vi "myRIO_BRig_Host_endExp_storeFiles__v4.vi"(0 "input_filePath":path) -> ()   [LabVIEW 2014]
panel:
  out "error2":errorcluster
  out "error1":errorcluster
  in  "input_error":errorcluster
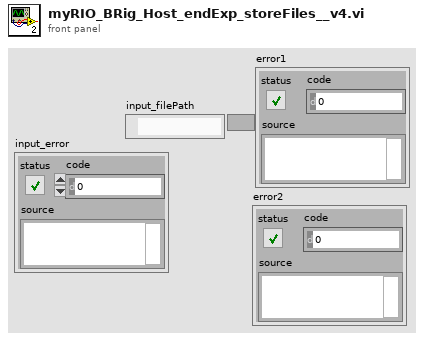
[diagram p1: front panel]
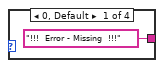
[diagram p2: hidden frame]
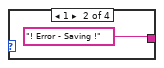
[diagram p3: hidden frame]
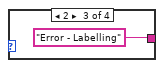
[diagram p4: hidden frame]
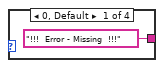
[diagram p5: hidden frame]
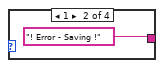
[diagram p6: hidden frame]
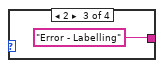
[diagram p7: hidden frame]
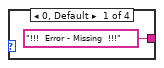
[diagram p8: hidden frame]
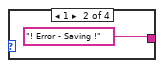
[diagram p9: hidden frame]
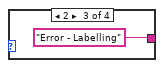
[diagram p10: hidden frame]
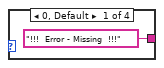
[diagram p11: hidden frame]
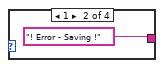
[diagram p12: hidden frame]
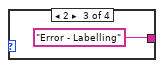
[diagram p13: hidden frame]
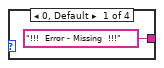
[diagram p14: hidden frame]
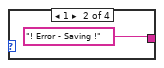
[diagram p15: hidden frame]
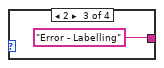
[diagram p16: hidden frame]
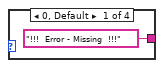
[diagram p17: hidden frame]
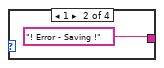
[diagram p18: hidden frame]
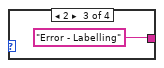
[diagram p19: hidden frame]
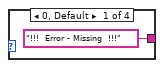
[diagram p20: hidden frame]
diagram:
  w2 = "\r"
  # "Workbooks"
  # "Application"
  # "Is Excel Running?"
  n1 = flat-sequence {
    tunnel: "input_filePath" -> [w403]
    tunnel: "input_error" -> [w400]
    tunnel: [w399] -> w395
    tunnel: [w402] -> w394
    tunnel: [w401] -> w393
    tunnel: [w398] -> w391
    tunnel: w395 -> [w446]
    tunnel: w394 -> [w447]
    tunnel: w393 -> [w407]
    tunnel: [w447] -> w392
    tunnel: w391 -> [w406]
    tunnel: [w446] -> w390
    tunnel: [w442] -> w389
    tunnel: [w441] -> w388
    tunnel: [w437] -> w314
    tunnel: [w436] -> w307
    tunnel: [w433] -> w279
    tunnel: [w430] -> w278
    tunnel: [w429] -> w277
    tunnel: [w428] -> w276
    tunnel: [w422] -> w268
    tunnel: [w421] -> w267
    tunnel: [w417] -> w266
    tunnel: [w416] -> w265
    tunnel: [w412] -> w264
    tunnel: [w411] -> w263
    tunnel: [w405] -> w40
    tunnel: [w404] -> w39
    tunnel: w392 -> [w489]
    tunnel: w390 -> [w485]
    tunnel: w389 -> [w484]
    tunnel: w388 -> [w488]
    tunnel: [w489] -> w387
    tunnel: [w487] -> w386
    tunnel: [w486] -> w385
    tunnel: [w450] -> w384
    tunnel: [w484] -> w383
    tunnel: [w483] -> w315
    tunnel: w314 -> [w483]
    tunnel: [w481] -> w308
    tunnel: w307 -> [w482]
    tunnel: [w480] -> w306
    tunnel: w279 -> [w478]
    tunnel: w278 -> [w477]
    tunnel: w277 -> [w465]
    tunnel: w276 -> [w467]
    tunnel: [w478] -> w270
    tunnel: w268 -> [w476]
    tunnel: w267 -> [w469]
    tunnel: w266 -> [w475]
    tunnel: w265 -> [w471]
    tunnel: w264 -> [w474]
    tunnel: w263 -> [w473]
    tunnel: [w464] -> w257
    tunnel: [w477] -> w251
    tunnel: [w466] -> w245
    tunnel: [w476] -> w239
    tunnel: [w468] -> w233
    tunnel: [w475] -> w227
    tunnel: [w470] -> w221
    tunnel: [w474] -> w215
    tunnel: [w472] -> w209
    tunnel: [w458] -> w208
    tunnel: [w457] -> w198
    tunnel: [w456] -> w190
    tunnel: [w455] -> w184
    tunnel: [w454] -> w179
    tunnel: [w453] -> w41
    tunnel: w40 -> [w453]
    tunnel: w39 -> [w452]
    tunnel: [w449] -> w38
    tunnel: [w448] -> w35
    tunnel: w387 -> [w531]
    tunnel: w386 -> [w529]
    tunnel: w385 -> [w528]
    tunnel: w384 -> [w495]
    tunnel: w383 -> [w530]
    tunnel: [w531] -> w370
    tunnel: [w530] -> w368
    tunnel: [w529] -> w366
    tunnel: [w528] -> w364
    tunnel: [w527] -> w362
    tunnel: [w522] -> w360
    tunnel: [w524] -> w316
    tunnel: w315 -> [w524]
    tunnel: [w525] -> w309
    tunnel: w308 -> [w525]
    tunnel: w306 -> [w526]
    tunnel: [w526] -> w305
    tunnel: [w523] -> w301
    tunnel: [w519] -> w271
    tunnel: w270 -> [w519]
    tunnel: [w520] -> w258
    tunnel: w257 -> [w520]
    tunnel: [w515] -> w252
    tunnel: w251 -> [w515]
    tunnel: [w516] -> w246
    tunnel: w245 -> [w516]
    tunnel: [w506] -> w240
    tunnel: w239 -> [w506]
    tunnel: [w509] -> w234
    tunnel: w233 -> [w509]
    tunnel: [w505] -> w228
    tunnel: w227 -> [w505]
    tunnel: [w508] -> w222
    tunnel: w221 -> [w508]
    tunnel: [w504] -> w216
    tunnel: w215 -> [w504]
    tunnel: [w507] -> w210
    tunnel: w209 -> [w507]
    tunnel: w208 -> [w521]
    tunnel: [w521] -> w204
    tunnel: [w518] -> w203
    tunnel: w198 -> [w517]
    tunnel: [w517] -> w196
    tunnel: [w514] -> w193
    tunnel: [w513] -> w191
    tunnel: w190 -> [w510]
    tunnel: [w510] -> w185
    tunnel: w184 -> [w511]
    tunnel: [w511] -> w180
    tunnel: w179 -> [w512]
    tunnel: [w512] -> w175
    tunnel: [w503] -> w174
    tunnel: [w502] -> w169
    tunnel: [w501] -> w164
    tunnel: [w500] -> w155
    tunnel: [w499] -> w153
    tunnel: [w498] -> w151
    tunnel: [w497] -> w149
    tunnel: [w496] -> w147
    tunnel: [w494] -> w42
    tunnel: w41 -> [w494]
    tunnel: w38 -> [w493]
    tunnel: [w493] -> w36
    tunnel: w35 -> [w492]
    tunnel: [w492] -> w33
    tunnel: [w491] -> w32
    tunnel: [w490] -> w31
    tunnel: w370 -> [w639]
    tunnel: [w639] -> w369
    tunnel: w368 -> [w638]
    tunnel: [w638] -> w367
    tunnel: w366 -> [w637]
    tunnel: [w637] -> w365
    tunnel: w364 -> [w636]
    tunnel: [w636] -> w363
    tunnel: w362 -> [w634]
    tunnel: [w634] -> w361
    tunnel: w360 -> [w635]
    tunnel: [w635] -> w359
    tunnel: [w630] -> w317
    tunnel: w316 -> [w630]
    tunnel: [w629] -> w310
    tunnel: w309 -> [w629]
    tunnel: w305 -> [w628]
    tunnel: [w628] -> w304
    tunnel: w301 -> [w627]
    tunnel: [w627] -> w300
    tunnel: [w626] -> w272
    tunnel: w271 -> [w626]
    tunnel: [w625] -> w259
    tunnel: w258 -> [w625]
    tunnel: [w624] -> w253
    tunnel: w252 -> [w624]
    tunnel: [w623] -> w247
    tunnel: w246 -> [w623]
    tunnel: [w622] -> w241
    tunnel: w240 -> [w622]
    tunnel: [w621] -> w235
    tunnel: w234 -> [w621]
    tunnel: [w620] -> w229
    tunnel: w228 -> [w620]
    tunnel: [w619] -> w223
    tunnel: w222 -> [w619]
    tunnel: [w618] -> w217
    tunnel: w216 -> [w618]
    tunnel: [w617] -> w211
    tunnel: w210 -> [w617]
    tunnel: [w616] -> w205
    tunnel: w204 -> [w616]
    tunnel: w203 -> [w615]
    tunnel: [w615] -> w199
    tunnel: [w614] -> w197
    tunnel: w196 -> [w614]
    tunnel: w193 -> [w606]
    tunnel: [w613] -> w192
    tunnel: w191 -> [w613]
    tunnel: [w612] -> w186
    tunnel: w185 -> [w612]
    tunnel: [w611] -> w181
    tunnel: w180 -> [w611]
    tunnel: [w610] -> w176
    tunnel: w175 -> [w610]
    tunnel: w174 -> [w609]
    tunnel: [w609] -> w170
    tunnel: w169 -> [w608]
    tunnel: [w608] -> w165
    tunnel: w164 -> [w607]
    tunnel: [w607] -> w160
    tunnel: [w606] -> w156
    tunnel: w155 -> [w605]
    tunnel: [w605] -> w154
    tunnel: w153 -> [w604]
    tunnel: [w604] -> w152
    tunnel: w151 -> [w603]
    tunnel: [w603] -> w150
    tunnel: w149 -> [w602]
    tunnel: [w602] -> w148
    tunnel: w147 -> [w601]
    tunnel: [w601] -> w146
    tunnel: [w600] -> w43
    tunnel: w42 -> [w600]
    tunnel: [w599] -> w37
    tunnel: w36 -> [w599]
    tunnel: [w598] -> w34
    tunnel: w33 -> [w598]
    tunnel: w32 -> [w596]
    tunnel: w31 -> [w597]
    tunnel: [w597] -> w30
    tunnel: [w596] -> w27
    tunnel: w369 -> [w704]
    tunnel: w367 -> [w703]
    tunnel: w365 -> [w701]
    tunnel: w363 -> [w700]
    tunnel: w361 -> [w702]
    tunnel: w359 -> [w697]
    tunnel: [w704] -> w382
    tunnel: [w703] -> w381
    tunnel: [w702] -> w380
    tunnel: [w684] -> w379
    tunnel: [w699] -> w378
    tunnel: [w698] -> w377
    tunnel: [w696] -> w318
    tunnel: w317 -> [w696]
    tunnel: [w692] -> w311
    tunnel: w310 -> [w694]
    tunnel: w304 -> [w693]
    tunnel: w300 -> [w695]
    tunnel: [w695] -> w299
    tunnel: [w691] -> w296
    tunnel: [w690] -> w273
    tunnel: w272 -> [w690]
    tunnel: [w651] -> w260
    tunnel: w259 -> [w677]
    tunnel: [w689] -> w254
    tunnel: w253 -> [w689]
    tunnel: [w654] -> w248
    tunnel: w247 -> [w674]
    tunnel: [w688] -> w242
    tunnel: w241 -> [w688]
    tunnel: [w657] -> w236
    tunnel: w235 -> [w671]
    tunnel: [w687] -> w230
    tunnel: w229 -> [w687]
    tunnel: [w660] -> w224
    tunnel: w223 -> [w668]
    tunnel: [w686] -> w218
    tunnel: w217 -> [w686]
    tunnel: [w663] -> w212
    tunnel: w211 -> [w678]
    tunnel: w205 -> [w676]
    tunnel: [w685] -> w200
    tunnel: w199 -> [w685]
    tunnel: w197 -> [w673]
    tunnel: w192 -> [w683]
    tunnel: [w662] -> w187
    tunnel: w186 -> [w665]
    tunnel: w181 -> [w667]
    tunnel: w176 -> [w670]
    tunnel: [w682] -> w171
    tunnel: w170 -> [w682]
    tunnel: [w681] -> w166
    tunnel: w165 -> [w681]
    tunnel: [w680] -> w161
    tunnel: w160 -> [w680]
    tunnel: [w679] -> w157
    tunnel: w156 -> [w679]
    tunnel: w154 -> [w675]
    tunnel: w152 -> [w672]
    tunnel: w150 -> [w669]
    tunnel: w148 -> [w666]
    tunnel: w146 -> [w664]
    tunnel: [w661] -> w145
    tunnel: [w659] -> w144
    tunnel: [w658] -> w143
    tunnel: [w656] -> w142
    tunnel: [w655] -> w141
    tunnel: [w653] -> w140
    tunnel: [w652] -> w139
    tunnel: [w650] -> w138
    tunnel: [w649] -> w137
    tunnel: [w648] -> w136
    tunnel: [w647] -> w44
    tunnel: w43 -> [w647]
    tunnel: w37 -> [w645]
    tunnel: w34 -> [w644]
    tunnel: w30 -> [w643]
    tunnel: [w646] -> w28
    tunnel: w27 -> [w646]
    tunnel: [w642] -> w24
    tunnel: [w641] -> w21
    tunnel: [w640] -> w18
    tunnel: w382 -> [w841]
    tunnel: w381 -> [w839]
    tunnel: w380 -> [w833]
    tunnel: w379 -> [w837]
    tunnel: w378 -> [w840]
    tunnel: w377 -> [w835]
    tunnel: [w841] -> w376
    tunnel: [w839] -> w375
    tunnel: [w838] -> w374
    tunnel: [w825] -> w373
    tunnel: [w840] -> w372
    tunnel: [w835] -> w371
    tunnel: [w831] -> w319
    tunnel: w318 -> [w831]
    tunnel: [w830] -> w312
    tunnel: w311 -> [w830]
    tunnel: [w826] -> w303
    tunnel: w299 -> [w828]
    tunnel: [w827] -> w298
    tunnel: w296 -> [w826]
    tunnel: [w816] -> w274
    tunnel: w273 -> [w816]
    tunnel: [w817] -> w261
    tunnel: w260 -> [w817]
    tunnel: [w809] -> w255
    tunnel: w254 -> [w809]
    tunnel: [w810] -> w249
    tunnel: w248 -> [w810]
    tunnel: [w801] -> w243
    tunnel: w242 -> [w801]
    tunnel: [w802] -> w237
    tunnel: w236 -> [w802]
    tunnel: [w788] -> w231
    tunnel: w230 -> [w788]
    tunnel: [w789] -> w225
    tunnel: w224 -> [w789]
    tunnel: [w782] -> w219
    tunnel: w218 -> [w782]
    tunnel: [w783] -> w213
    tunnel: w212 -> [w783]
    tunnel: [w819] -> w206
    tunnel: [w821] -> w201
    tunnel: w200 -> [w822]
    tunnel: [w813] -> w194
    tunnel: [w790] -> w188
    tunnel: w187 -> [w790]
    tunnel: [w791] -> w182
    tunnel: [w792] -> w177
    tunnel: [w778] -> w172
    tunnel: w171 -> [w780]
    tunnel: [w785] -> w167
    tunnel: w166 -> [w784]
    tunnel: [w798] -> w162
    tunnel: w161 -> [w799]
    tunnel: [w807] -> w158
    tunnel: w157 -> [w806]
    tunnel: w145 -> [w781]
    tunnel: w144 -> [w791]
    tunnel: w143 -> [w787]
    tunnel: w142 -> [w792]
    tunnel: w141 -> [w800]
    tunnel: w140 -> [w813]
    tunnel: w139 -> [w808]
    tunnel: w138 -> [w819]
    tunnel: w137 -> [w815]
    tunnel: w136 -> [w824]
    tunnel: [w823] -> w134
    tunnel: [w814] -> w132
    tunnel: [w805] -> w130
    tunnel: [w797] -> w128
    tunnel: [w786] -> w126
    tunnel: [w779] -> w124
    tunnel: [w771] -> w45
    tunnel: w44 -> [w771]
    tunnel: w28 -> [w773]
    tunnel: [w770] -> w25
    tunnel: w24 -> [w770]
    tunnel: [w772] -> w22
    tunnel: w21 -> [w772]
    tunnel: [w775] -> w19
    tunnel: w18 -> [w776]
    tunnel: [w774] -> w17
    tunnel: w376 -> [w941]
    tunnel: w375 -> [w946]
    tunnel: w374 -> [w945]
    tunnel: w373 -> [w944]
    tunnel: w372 -> [w943]
    tunnel: w371 -> [w942]
    tunnel: [w941] -> w358
    tunnel: [w946] -> w357
    tunnel: [w945] -> w356
    tunnel: [w944] -> w355
    tunnel: [w943] -> w354
    tunnel: [w942] -> w353
    tunnel: [w940] -> w320
    tunnel: w319 -> [w940]
    tunnel: [w939] -> w313
    tunnel: w312 -> [w939]
    tunnel: w303 -> [w938]
    tunnel: [w938] -> w302
    tunnel: w298 -> [w937]
    tunnel: [w937] -> w297
    tunnel: [w936] -> w275
    tunnel: w274 -> [w936]
    tunnel: [w935] -> w262
    tunnel: w261 -> [w935]
    tunnel: [w934] -> w256
    tunnel: w255 -> [w934]
    tunnel: [w933] -> w250
    tunnel: w249 -> [w933]
    tunnel: [w932] -> w244
    tunnel: w243 -> [w932]
    tunnel: [w931] -> w238
    tunnel: w237 -> [w931]
    tunnel: [w930] -> w232
    tunnel: w231 -> [w930]
    tunnel: [w929] -> w226
    tunnel: w225 -> [w929]
    tunnel: [w928] -> w220
    tunnel: w219 -> [w928]
    tunnel: [w927] -> w214
    tunnel: w213 -> [w927]
    tunnel: [w926] -> w207
    tunnel: w206 -> [w926]
    tunnel: [w925] -> w202
    tunnel: w201 -> [w925]
    tunnel: [w924] -> w195
    tunnel: w194 -> [w924]
    tunnel: [w923] -> w189
    tunnel: w188 -> [w923]
    tunnel: [w922] -> w183
    tunnel: w182 -> [w922]
    tunnel: [w921] -> w178
    tunnel: w177 -> [w921]
    tunnel: [w920] -> w173
    tunnel: w172 -> [w920]
    tunnel: [w919] -> w168
    tunnel: w167 -> [w919]
    tunnel: [w918] -> w163
    tunnel: w162 -> [w918]
    tunnel: [w917] -> w159
    tunnel: w158 -> [w917]
    tunnel: [w916] -> w135
    tunnel: w134 -> [w916]
    tunnel: [w915] -> w133
    tunnel: w132 -> [w915]
    tunnel: [w914] -> w131
    tunnel: w130 -> [w914]
    tunnel: [w913] -> w129
    tunnel: w128 -> [w913]
    tunnel: [w912] -> w127
    tunnel: w126 -> [w912]
    tunnel: [w911] -> w125
    tunnel: w124 -> [w911]
    tunnel: [w910] -> w46
    tunnel: w45 -> [w910]
    tunnel: [w909] -> w29
    tunnel: [w908] -> w26
    tunnel: w25 -> [w908]
    tunnel: [w907] -> w23
    tunnel: w22 -> [w907]
    tunnel: [w906] -> w20
    tunnel: w19 -> [w906]
    tunnel: w17 -> [w909]
    tunnel: w358 -> [w990]
    tunnel: w357 -> [w998]
    tunnel: w356 -> [w997]
    tunnel: w355 -> [w996]
    tunnel: w354 -> [w995]
    tunnel: w353 -> [w994]
    tunnel: [w990] -> w350
    tunnel: [w998] -> w346
    tunnel: [w997] -> w345
    tunnel: [w996] -> w342
    tunnel: [w995] -> w344
    tunnel: [w994] -> w343
    tunnel: [w986] -> w349
    tunnel: [w985] -> w348
    tunnel: [w984] -> w347
    tunnel: [w983] -> w295
    tunnel: w320 -> [w983]
    tunnel: [w982] -> w293
    tunnel: w313 -> [w982]
    tunnel: w302 -> [w981]
    tunnel: [w981] -> w292
    tunnel: w297 -> [w980]
    tunnel: [w980] -> w294
    tunnel: [w979] -> w269
    tunnel: w275 -> [w979]
    tunnel: [w978] -> w122
    tunnel: w262 -> [w978]
    tunnel: [w977] -> w120
    tunnel: w256 -> [w977]
    tunnel: [w976] -> w118
    tunnel: w250 -> [w976]
    tunnel: [w975] -> w116
    tunnel: w244 -> [w975]
    tunnel: [w974] -> w114
    tunnel: w238 -> [w974]
    tunnel: [w973] -> w112
    tunnel: w232 -> [w973]
    tunnel: [w972] -> w110
    tunnel: w226 -> [w972]
    tunnel: [w971] -> w108
    tunnel: w220 -> [w971]
    tunnel: [w970] -> w106
    tunnel: w214 -> [w970]
    tunnel: [w969] -> w121
    tunnel: w207 -> [w969]
    tunnel: [w968] -> w123
    tunnel: w202 -> [w968]
    tunnel: [w967] -> w117
    tunnel: w195 -> [w967]
    tunnel: [w966] -> w105
    tunnel: w189 -> [w966]
    tunnel: [w965] -> w109
    tunnel: w183 -> [w965]
    tunnel: [w964] -> w113
    tunnel: w178 -> [w964]
    tunnel: [w963] -> w107
    tunnel: w173 -> [w963]
    tunnel: [w962] -> w111
    tunnel: w168 -> [w962]
    tunnel: [w961] -> w115
    tunnel: w163 -> [w961]
    tunnel: [w960] -> w119
    tunnel: w159 -> [w960]
    tunnel: [w959] -> w104
    tunnel: w135 -> [w959]
    tunnel: [w958] -> w103
    tunnel: w133 -> [w958]
    tunnel: [w957] -> w102
    tunnel: w131 -> [w957]
    tunnel: [w956] -> w101
    tunnel: w129 -> [w956]
    tunnel: [w955] -> w100
    tunnel: w127 -> [w955]
    tunnel: [w954] -> w99
    tunnel: w125 -> [w954]
    tunnel: w46 -> [w953]
    tunnel: [w953] -> w16
    tunnel: [w952] -> w15
    tunnel: w29 -> [w952]
    tunnel: [w951] -> w14
    tunnel: w26 -> [w951]
    tunnel: [w950] -> w13
    tunnel: w23 -> [w950]
    tunnel: [w949] -> w12
    tunnel: w20 -> [w949]
    frame #0 {
      # "Is Excel Running?"
      # "Prepare storage"
      # "get Exp Prefix"
      n2 = call "myRIO_BRig_Host_endExp_getExp.vi"("input_filePath"=w403) -> ("output_expPrefix"=w401:string)  [unwired: 10 in]
      n3 = call "myRIO_BRig_Host_isExcelRunning.vi"() -> ("output_Iexcel"=w402:bool)  [unwired: 11 in]
      n4 = call "myRIO_BRig_Host_endExp_prepareStoreLocation.vi"("input_error"=w400, "input_expPrefix"=w401) -> ("output_error"=w399:errorcluster, "output_folderPath"=w398:string)  [unwired: 8 in]
    }
    frame #1 {
      w408 = "dataAnalog" ("input_fileName")
      w413 = "dataTrial" ("input_fileName")
      w418 = "dataMTrig" ("input_fileName")
      w423 = "dataLick" ("input_fileName")
      w427 = "dataLC" ("input_fileName")
      w426 = "dataExp" ("input_fileName")
      w438 = "dataCurrent" ("input_fileName")
      w445 = "dataBlock" ("input_fileName")
      # "original"
      # "storage"
      # "original"
      # "storage"
      # "original"
      # "storage"
      # "original"
      # "storage"
      # "original"
      # "storage"
      # "original"
      # "storage"
      # "original"
      # "storage"
      # "original"
      # "storage"
      # "Prepare file paths"
      n5 = call "myRIO_BRig_Host_endExp_filePath__originalLocation.vi"("input_expPrefix"=w407, "input_fileName"=w426) -> ("output_filePath"=w434:string)  [unwired: 9 in]
      n6 = call "myRIO_BRig_Host_endExp_filePath__storeLocation.vi"("input_expPrefix"=w407, "input_fileName"=w426, "input_filePath_storage"=w406) -> ("output_filePath"=w435:string)  [unwired: 8 in]
      n7 = call "myRIO_BRig_Host_endExp_filePath__originalLocation.vi"("input_expPrefix"=w407, "input_fileName"=w413) -> ("output_filePath"=w414:string)  [unwired: 9 in]
      n8 = call "myRIO_BRig_Host_endExp_filePath__originalLocation.vi"("input_expPrefix"=w407, "input_fileName"=w438) -> ("output_filePath"=w439:string)  [unwired: 9 in]
      n9 = call "myRIO_BRig_Host_endExp_filePath__originalLocation.vi"("input_expPrefix"=w407, "input_fileName"=w427) -> ("output_filePath"=w431:string)  [unwired: 9 in]
      n10 = call "myRIO_BRig_Host_endExp_filePath__originalLocation.vi"("input_expPrefix"=w407, "input_fileName"=w423) -> ("output_filePath"=w424:string)  [unwired: 9 in]
      n11 = call "myRIO_BRig_Host_endExp_filePath__originalLocation.vi"("input_expPrefix"=w407, "input_fileName"=w418) -> ("output_filePath"=w419:string)  [unwired: 9 in]
      n12 = call "myRIO_BRig_Host_endExp_filePath__storeLocation.vi"("input_expPrefix"=w407, "input_fileName"=w413, "input_filePath_storage"=w406) -> ("output_filePath"=w415:string)  [unwired: 8 in]
      n13 = call "myRIO_BRig_Host_endExp_filePath__originalLocation.vi"("input_expPrefix"=w407, "input_fileName"=w408) -> ("output_filePath"=w409:string)  [unwired: 9 in]
      n14 = call "myRIO_BRig_Host_endExp_filePath__storeLocation.vi"("input_expPrefix"=w407, "input_fileName"=w438, "input_filePath_storage"=w406) -> ("output_filePath"=w440:string)  [unwired: 8 in]
      n15 = call "myRIO_BRig_Host_endExp_filePath__storeLocation.vi"("input_expPrefix"=w407, "input_fileName"=w427, "input_filePath_storage"=w406) -> ("output_filePath"=w432:string)  [unwired: 8 in]
      n16 = call "myRIO_BRig_Host_endExp_filePath__storeLocation.vi"("input_expPrefix"=w407, "input_fileName"=w423, "input_filePath_storage"=w406) -> ("output_filePath"=w425:string)  [unwired: 8 in]
      n17 = call "myRIO_BRig_Host_endExp_filePath__storeLocation.vi"("input_expPrefix"=w407, "input_fileName"=w418, "input_filePath_storage"=w406) -> ("output_filePath"=w420:string)  [unwired: 8 in]
      n18 = call "myRIO_BRig_Host_endExp_filePath__storeLocation.vi"("input_expPrefix"=w407, "input_fileName"=w408, "input_filePath_storage"=w406) -> ("output_filePath"=w410:string)  [unwired: 8 in]
      n19 = call "myRIO_BRig_Host_endExp_filePath__originalLocation.vi"("input_expPrefix"=w407, "input_fileName"=w445) -> ("output_filePath"=w443:string)  [unwired: 9 in]
      n20 = call "myRIO_BRig_Host_endExp_filePath__storeLocation.vi"("input_expPrefix"=w407, "input_fileName"=w445, "input_filePath_storage"=w406) -> ("output_filePath"=w444:string)  [unwired: 8 in]
      n21 = String To Path(string=w435) -> (path=w433:path)
      n22 = String To Path(string=w434) -> (path=w429:path)
      n23 = String To Path(string=w415) -> (path=w412:path)
      n24 = String To Path(string=w414) -> (path=w411:path)
      n25 = String To Path(string=w440) -> (path=w437:path)
      n26 = String To Path(string=w439) -> (path=w436:path)
      n27 = String To Path(string=w432) -> (path=w430:path)
      n28 = String To Path(string=w431) -> (path=w428:path)
      n29 = String To Path(string=w425) -> (path=w422:path)
      n30 = String To Path(string=w424) -> (path=w421:path)
      n31 = String To Path(string=w420) -> (path=w417:path)
      n32 = String To Path(string=w419) -> (path=w416:path)
      n33 = String To Path(string=w410) -> (path=w405:path)
      n34 = String To Path(string=w409) -> (path=w404:path)
      n35 = String To Path(string=w444) -> (path=w442:path)
      n36 = String To Path(string=w443) -> (path=w441:path)
    }
    frame #2 {
      # "Check if\noriginal files\nexist"
      n37 = call "myRIO_BRig_generic_pathExists_fast_pathInput.vi"("input_error"=w485, "input_filePath"=w488) -> ("output_error"=w479:errorcluster, "output_Iexist"=w486:bool, "output_filePath"=w487:path)  [unwired: 7 in]
      n38 = call "myRIO_BRig_generic_pathExists_fast_pathInput.vi"("input_error"=w479, "input_filePath"=w482) -> ("output_error"=w463:errorcluster, "output_Iexist"=w480:bool, "output_filePath"=w481:path)  [unwired: 7 in]
      n39 = call "myRIO_BRig_generic_pathExists_fast_pathInput.vi"("input_error"=w463, "input_filePath"=w465) -> ("output_error"=w462:errorcluster, "output_Iexist"=w458:bool, "output_filePath"=w464:path)  [unwired: 7 in]
      n40 = call "myRIO_BRig_generic_pathExists_fast_pathInput.vi"("input_error"=w462, "input_filePath"=w467) -> ("output_error"=w461:errorcluster, "output_Iexist"=w457:bool, "output_filePath"=w466:path)  [unwired: 7 in]
      n41 = call "myRIO_BRig_generic_pathExists_fast_pathInput.vi"("input_error"=w461, "input_filePath"=w469) -> ("output_error"=w460:errorcluster, "output_Iexist"=w454:bool, "output_filePath"=w468:path)  [unwired: 7 in]
      n42 = call "myRIO_BRig_generic_pathExists_fast_pathInput.vi"("input_error"=w460, "input_filePath"=w471) -> ("output_error"=w459:errorcluster, "output_Iexist"=w455:bool, "output_filePath"=w470:path)  [unwired: 7 in]
      n43 = call "myRIO_BRig_generic_pathExists_fast_pathInput.vi"("input_error"=w459, "input_filePath"=w473) -> ("output_error"=w451:errorcluster, "output_Iexist"=w456:bool, "output_filePath"=w472:path)  [unwired: 7 in]
      n44 = call "myRIO_BRig_generic_pathExists_fast_pathInput.vi"("input_error"=w451, "input_filePath"=w452) -> ("output_error"=w450:errorcluster, "output_Iexist"=w448:bool, "output_filePath"=w449:path)  [unwired: 7 in]
    }
    frame #3 {
      # "If original files exist,\nthen store them"
      n45 = case shown="True" w528 {
        selector: w528 -> [w588 w593]
        tunnel: w529 -> [_ w595]
        tunnel: w530 -> [_ w594]
        tunnel: w495 -> [w589 w592]
        tunnel: [w589 w591] -> w522
        tunnel: [w588 w590] -> w527
        frame False {
        }
        frame True {
          n46 = call "myRIO_BRig_generic_pathMove_pathInput.vi"("input_error"=w592, "input_Ioverwrite"=w593, "input_filePath_target"=w594, "input_filePath_source"=w595) -> ("output_error"=w591:errorcluster, "output_Iexist"=w590:bool)  [unwired: 5 in, 1 out]
        }
      }
      n47 = case shown="True" w526 {
        selector: w526 -> [w580 w585]
        tunnel: w525 -> [_ w587]
        tunnel: w524 -> [_ w586]
        tunnel: w495 -> [w581 w584]
        tunnel: [w581 w583] -> w513
        tunnel: [w580 w582] -> w523
        frame False {
        }
        frame True {
          n48 = call "myRIO_BRig_generic_pathMove_pathInput.vi"("input_error"=w584, "input_Ioverwrite"=w585, "input_filePath_target"=w586, "input_filePath_source"=w587) -> ("output_error"=w583:errorcluster, "output_Iexist"=w582:bool)  [unwired: 5 in, 1 out]
        }
      }
      n49 = case shown="True" w521 {
        selector: w521 -> [w572 w577]
        tunnel: w520 -> [_ w579]
        tunnel: w519 -> [_ w578]
        tunnel: w495 -> [w573 w576]
        tunnel: [w573 w575] -> w500
        tunnel: [w572 w574] -> w518
        frame False {
        }
        frame True {
          n50 = call "myRIO_BRig_generic_pathMove_pathInput.vi"("input_error"=w576, "input_Ioverwrite"=w577, "input_filePath_target"=w578, "input_filePath_source"=w579) -> ("output_error"=w575:errorcluster, "output_Iexist"=w574:bool)  [unwired: 5 in, 1 out]
        }
      }
      n51 = case shown="True" w517 {
        selector: w517 -> [w564 w569]
        tunnel: w516 -> [_ w571]
        tunnel: w515 -> [_ w570]
        tunnel: w495 -> [w565 w568]
        tunnel: [w565 w567] -> w499
        tunnel: [w564 w566] -> w514
        frame False {
        }
        frame True {
          n52 = call "myRIO_BRig_generic_pathMove_pathInput.vi"("input_error"=w568, "input_Ioverwrite"=w569, "input_filePath_target"=w570, "input_filePath_source"=w571) -> ("output_error"=w567:errorcluster, "output_Iexist"=w566:bool)  [unwired: 5 in, 1 out]
        }
      }
      n53 = case shown="True" w512 {
        selector: w512 -> [w556 w561]
        tunnel: w509 -> [_ w563]
        tunnel: w506 -> [_ w562]
        tunnel: w495 -> [w557 w560]
        tunnel: [w557 w559] -> w498
        tunnel: [w556 w558] -> w501
        frame False {
        }
        frame True {
          n54 = call "myRIO_BRig_generic_pathMove_pathInput.vi"("input_error"=w560, "input_Ioverwrite"=w561, "input_filePath_target"=w562, "input_filePath_source"=w563) -> ("output_error"=w559:errorcluster, "output_Iexist"=w558:bool)  [unwired: 5 in, 1 out]
        }
      }
      n55 = case shown="True" w511 {
        selector: w511 -> [w548 w553]
        tunnel: w508 -> [_ w555]
        tunnel: w505 -> [_ w554]
        tunnel: w495 -> [w549 w552]
        tunnel: [w549 w551] -> w497
        tunnel: [w548 w550] -> w502
        frame False {
        }
        frame True {
          n56 = call "myRIO_BRig_generic_pathMove_pathInput.vi"("input_error"=w552, "input_Ioverwrite"=w553, "input_filePath_target"=w554, "input_filePath_source"=w555) -> ("output_error"=w551:errorcluster, "output_Iexist"=w550:bool)  [unwired: 5 in, 1 out]
        }
      }
      n57 = case shown="True" w510 {
        selector: w510 -> [w540 w545]
        tunnel: w507 -> [_ w547]
        tunnel: w504 -> [_ w546]
        tunnel: w495 -> [w541 w544]
        tunnel: [w541 w543] -> w496
        tunnel: [w540 w542] -> w503
        frame False {
        }
        frame True {
          n58 = call "myRIO_BRig_generic_pathMove_pathInput.vi"("input_error"=w544, "input_Ioverwrite"=w545, "input_filePath_target"=w546, "input_filePath_source"=w547) -> ("output_error"=w543:errorcluster, "output_Iexist"=w542:bool)  [unwired: 5 in, 1 out]
        }
      }
      n59 = case shown="True" w492 {
        selector: w492 -> [w532 w537]
        tunnel: w493 -> [_ w539]
        tunnel: w494 -> [_ w538]
        tunnel: w495 -> [w533 w536]
        tunnel: [w533 w535] -> w490
        tunnel: [w532 w534] -> w491
        frame False {
        }
        frame True {
          n60 = call "myRIO_BRig_generic_pathMove_pathInput.vi"("input_error"=w536, "input_Ioverwrite"=w537, "input_filePath_target"=w538, "input_filePath_source"=w539) -> ("output_error"=w535:errorcluster, "output_Iexist"=w534:bool)  [unwired: 5 in, 1 out]
        }
      }
    }
    frame #4 {
      # "Add a delay\nin case\nall files\nweren't stored"
      n61 = Select(t=u32 0 ("milliseconds to wait"), s=w634, f=u32 200 ("milliseconds to wait")) -> (s? t:f=w633:u32)
      n62 = Wait (ms)(milliseconds to wait=w633) -> ()  [unwired: 1 out]
    }
    frame #5 {
      # "Re-check\noriginal files"
      n63 = case shown="False" w700 {
        selector: w700 -> [_ w767]
        tunnel: w701 -> [w765 w768]
        tunnel: w697 -> [w764 w766]
        tunnel: [w763 w766] -> w684
        tunnel: [w762 w768] -> w699
        tunnel: [w761 w767] -> w698
        frame False {
          n64 = call "myRIO_BRig_generic_pathExists_fast_pathInput.vi"("input_error"=w764, "input_filePath"=w765) -> ("output_error"=w763:errorcluster, "output_Iexist"=w761:bool, "output_filePath"=w762:path)  [unwired: 7 in]
        }
        frame True {
        }
      }
      n65 = case shown="False" w693 {
        selector: w693 -> [_ w759]
        tunnel: w694 -> [w757 w760]
        tunnel: w683 -> [w756 w758]
        tunnel: [w755 w758] -> w648
        tunnel: [w754 w760] -> w692
        tunnel: [w753 w759] -> w691
        frame False {
          n66 = call "myRIO_BRig_generic_pathExists_fast_pathInput.vi"("input_error"=w756, "input_filePath"=w757) -> ("output_error"=w755:errorcluster, "output_Iexist"=w753:bool, "output_filePath"=w754:path)  [unwired: 7 in]
        }
        frame True {
        }
      }
      n67 = case shown="False" w676 {
        selector: w676 -> [_ w751]
        tunnel: w677 -> [w749 w752]
        tunnel: w675 -> [w748 w750]
        tunnel: [w747 w750] -> w649
        tunnel: [w746 w752] -> w651
        tunnel: [w745 w751] -> w650
        frame False {
          n68 = call "myRIO_BRig_generic_pathExists_fast_pathInput.vi"("input_error"=w748, "input_filePath"=w749) -> ("output_error"=w747:errorcluster, "output_Iexist"=w745:bool, "output_filePath"=w746:path)  [unwired: 7 in]
        }
        frame True {
        }
      }
      n69 = case shown="False" w673 {
        selector: w673 -> [_ w743]
        tunnel: w674 -> [w741 w744]
        tunnel: w672 -> [w740 w742]
        tunnel: [w739 w742] -> w652
        tunnel: [w738 w744] -> w654
        tunnel: [w737 w743] -> w653
        frame False {
          n70 = call "myRIO_BRig_generic_pathExists_fast_pathInput.vi"("input_error"=w740, "input_filePath"=w741) -> ("output_error"=w739:errorcluster, "output_Iexist"=w737:bool, "output_filePath"=w738:path)  [unwired: 7 in]
        }
        frame True {
        }
      }
      n71 = case shown="False" w670 {
        selector: w670 -> [_ w735]
        tunnel: w671 -> [w733 w736]
        tunnel: w669 -> [w732 w734]
        tunnel: [w731 w734] -> w655
        tunnel: [w730 w736] -> w657
        tunnel: [w729 w735] -> w656
        frame False {
          n72 = call "myRIO_BRig_generic_pathExists_fast_pathInput.vi"("input_error"=w732, "input_filePath"=w733) -> ("output_error"=w731:errorcluster, "output_Iexist"=w729:bool, "output_filePath"=w730:path)  [unwired: 7 in]
        }
        frame True {
        }
      }
      n73 = case shown="False" w667 {
        selector: w667 -> [_ w727]
        tunnel: w668 -> [w725 w728]
        tunnel: w666 -> [w724 w726]
        tunnel: [w723 w726] -> w658
        tunnel: [w722 w728] -> w660
        tunnel: [w721 w727] -> w659
        frame False {
          n74 = call "myRIO_BRig_generic_pathExists_fast_pathInput.vi"("input_error"=w724, "input_filePath"=w725) -> ("output_error"=w723:errorcluster, "output_Iexist"=w721:bool, "output_filePath"=w722:path)  [unwired: 7 in]
        }
        frame True {
        }
      }
      n75 = case shown="False" w665 {
        selector: w665 -> [_ w719]
        tunnel: w678 -> [w717 w720]
        tunnel: w664 -> [w716 w718]
        tunnel: [w715 w718] -> w661
        tunnel: [w714 w720] -> w663
        tunnel: [w713 w719] -> w662
        frame False {
          n76 = call "myRIO_BRig_generic_pathExists_fast_pathInput.vi"("input_error"=w716, "input_filePath"=w717) -> ("output_error"=w715:errorcluster, "output_Iexist"=w713:bool, "output_filePath"=w714:path)  [unwired: 7 in]
        }
        frame True {
        }
      }
      n77 = case shown="False" w644 {
        selector: w644 -> [_ w711]
        tunnel: w645 -> [w709 w712]
        tunnel: w643 -> [w708 w710]
        tunnel: [w707 w710] -> w640
        tunnel: [w706 w712] -> w642
        tunnel: [w705 w711] -> w641
        frame False {
          n78 = call "myRIO_BRig_generic_pathExists_fast_pathInput.vi"("input_error"=w708, "input_filePath"=w709) -> ("output_error"=w707:errorcluster, "output_Iexist"=w705:bool, "output_filePath"=w706:path)  [unwired: 7 in]
        }
        frame True {
        }
      }
    }
    frame #6 {
      # "Re-check\nstorage"
      n79 = Not(x=w833) -> (.not. x?=w836:bool)
      n80 = Not(x=w828) -> (.not. x?=w832:bool)
      n81 = Not(x=w799) -> (.not. x?=w803:bool)
      n82 = Not(x=w784) -> (.not. x?=w796:bool)
      n83 = Not(x=w806) -> (.not. x?=w812:bool)
      n84 = Not(x=w780) -> (.not. x?=w793:bool)
      n85 = Not(x=w773) -> (.not. x?=w777:bool)
      n86 = Not(x=w822) -> (.not. x?=w820:bool)
      n87 = And(x=w836, y=w835) -> (x .and. y?=w834:bool)
      n88 = And(x=w832, y=w826) -> (x .and. y?=w829:bool)
      n89 = And(x=w803, y=w792) -> (x .and. y?=w804:bool)
      n90 = And(x=w796, y=w791) -> (x .and. y?=w795:bool)
      n91 = And(x=w812, y=w813) -> (x .and. y?=w811:bool)
      n92 = And(x=w793, y=w790) -> (x .and. y?=w794:bool)
      n93 = And(x=w777, y=w772) -> (x .and. y?=w769:bool)
      n94 = And(x=w820, y=w819) -> (x .and. y?=w818:bool)
      n95 = case shown="True" w834 {
        selector: w834 -> [_ w903]
        tunnel: w840 -> [_ w905]
        tunnel: w839 -> [_ w904]
        tunnel: w837 -> [w899 w902]
        tunnel: [w899 w901] -> w825
        tunnel: [w898 w900] -> w838
        tunnel: w833 -> [w898 _]
        frame False {
        }
        frame True {
          n96 = call "myRIO_BRig_generic_pathMove_pathInput.vi"("input_error"=w902, "input_Ioverwrite"=w903, "input_filePath_target"=w904, "input_filePath_source"=w905) -> ("output_error"=w901:errorcluster, "output_Iexist"=w900:bool)  [unwired: 5 in, 1 out]
        }
      }
      n97 = case shown="True" w829 {
        selector: w829 -> [_ w895]
        tunnel: w830 -> [_ w897]
        tunnel: w831 -> [_ w896]
        tunnel: w824 -> [w891 w894]
        tunnel: [w891 w893] -> w823
        tunnel: [w890 w892] -> w827
        tunnel: w828 -> [w890 _]
        frame False {
        }
        frame True {
          n98 = call "myRIO_BRig_generic_pathMove_pathInput.vi"("input_error"=w894, "input_Ioverwrite"=w895, "input_filePath_target"=w896, "input_filePath_source"=w897) -> ("output_error"=w893:errorcluster, "output_Iexist"=w892:bool)  [unwired: 5 in, 1 out]
        }
      }
      n99 = case shown="True" w818 {
        selector: w818 -> [_ w887]
        tunnel: w817 -> [_ w889]
        tunnel: w816 -> [_ w888]
        tunnel: w815 -> [w883 w886]
        tunnel: [w883 w885] -> w814
        tunnel: [w882 w884] -> w821
        tunnel: w822 -> [w882 _]
        frame False {
        }
        frame True {
          n100 = call "myRIO_BRig_generic_pathMove_pathInput.vi"("input_error"=w886, "input_Ioverwrite"=w887, "input_filePath_target"=w888, "input_filePath_source"=w889) -> ("output_error"=w885:errorcluster, "output_Iexist"=w884:bool)  [unwired: 5 in, 1 out]
        }
      }
      n101 = case shown="True" w811 {
        selector: w811 -> [_ w879]
        tunnel: w810 -> [_ w881]
        tunnel: w809 -> [_ w880]
        tunnel: w808 -> [w875 w878]
        tunnel: [w875 w877] -> w805
        tunnel: [w874 w876] -> w807
        tunnel: w806 -> [w874 _]
        frame False {
        }
        frame True {
          n102 = call "myRIO_BRig_generic_pathMove_pathInput.vi"("input_error"=w878, "input_Ioverwrite"=w879, "input_filePath_target"=w880, "input_filePath_source"=w881) -> ("output_error"=w877:errorcluster, "output_Iexist"=w876:bool)  [unwired: 5 in, 1 out]
        }
      }
      n103 = case shown="True" w804 {
        selector: w804 -> [_ w871]
        tunnel: w802 -> [_ w873]
        tunnel: w801 -> [_ w872]
        tunnel: w800 -> [w867 w870]
        tunnel: [w867 w869] -> w797
        tunnel: [w866 w868] -> w798
        tunnel: w799 -> [w866 _]
        frame False {
        }
        frame True {
          n104 = call "myRIO_BRig_generic_pathMove_pathInput.vi"("input_error"=w870, "input_Ioverwrite"=w871, "input_filePath_target"=w872, "input_filePath_source"=w873) -> ("output_error"=w869:errorcluster, "output_Iexist"=w868:bool)  [unwired: 5 in, 1 out]
        }
      }
      n105 = case shown="True" w795 {
        selector: w795 -> [_ w863]
        tunnel: w789 -> [_ w865]
        tunnel: w788 -> [_ w864]
        tunnel: w787 -> [w859 w862]
        tunnel: [w859 w861] -> w786
        tunnel: [w858 w860] -> w785
        tunnel: w784 -> [w858 _]
        frame False {
        }
        frame True {
          n106 = call "myRIO_BRig_generic_pathMove_pathInput.vi"("input_error"=w862, "input_Ioverwrite"=w863, "input_filePath_target"=w864, "input_filePath_source"=w865) -> ("output_error"=w861:errorcluster, "output_Iexist"=w860:bool)  [unwired: 5 in, 1 out]
        }
      }
      n107 = case shown="True" w794 {
        selector: w794 -> [_ w855]
        tunnel: w783 -> [_ w857]
        tunnel: w782 -> [_ w856]
        tunnel: w781 -> [w851 w854]
        tunnel: [w851 w853] -> w779
        tunnel: [w850 w852] -> w778
        tunnel: w780 -> [w850 _]
        frame False {
        }
        frame True {
          n108 = call "myRIO_BRig_generic_pathMove_pathInput.vi"("input_error"=w854, "input_Ioverwrite"=w855, "input_filePath_target"=w856, "input_filePath_source"=w857) -> ("output_error"=w853:errorcluster, "output_Iexist"=w852:bool)  [unwired: 5 in, 1 out]
        }
      }
      n109 = case shown="True" w769 {
        selector: w769 -> [_ w847]
        tunnel: w770 -> [_ w849]
        tunnel: w771 -> [_ w848]
        tunnel: w776 -> [w843 w846]
        tunnel: [w843 w845] -> w775
        tunnel: [w842 w844] -> w774
        tunnel: w773 -> [w842 _]
        frame False {
        }
        frame True {
          n110 = call "myRIO_BRig_generic_pathMove_pathInput.vi"("input_error"=w846, "input_Ioverwrite"=w847, "input_filePath_target"=w848, "input_filePath_source"=w849) -> ("output_error"=w845:errorcluster, "output_Iexist"=w844:bool)  [unwired: 5 in, 1 out]
        }
      }
    }
    frame #7 {
      # "Check if Excel\nis running"
      n111 = case shown="True" w941 {
        frame False {
        }
        frame True {
          n112 = One Button Dialog(message="!!! Warning !!!  Save all Excel work, then press okay\n(If Excel isn't visible, use Ctrl-Alt-Delete)", button name ("OK")="I have saved any Excel work") -> ()  [unwired: 1 out]
        }
      }
    }
    frame #8 {
      w993 = refnum<k7> refnum  # Excel._Application
      # "Is Excel Running?"
      # "Open Excel via LabView"
      # "Workbooks"
      # "Application"
      n113 = Automation Open(Automation Refnum=w993) -> (Automation Refnum=w992:refnum<k7>, error out=w991:errorcluster)  [unwired: 1 in, 2 out]
      n114 = case shown="False" w990 {
        tunnel: w992 -> [w1002 w1005]
        tunnel: w991 -> [w1001 w1004]
        tunnel: [w1000 w1004] -> w988
        tunnel: [w999 w1005] -> w987
        frame False {
          n115 = property class="_Application"(reference=w1002, error in=w1001, "Visible"=FALSE) -> (reference out=w999:refnum<k7>, error out=w1000:errorcluster)
        }
        frame True {
        }
      }
      n116 = property class="_Application"(reference=w987, error in=w988, "DisplayAlerts"=FALSE) -> (reference out=w985:refnum<k7>, error out=w986:errorcluster, "Workbooks"=w984:refnum<k7>)
    }
  }
  n117 = Unbundle By Name(w349) -> ("code"=w352:i32)
  n118 = Equal To 0?(x=w352) -> (x = 0?=w351:bool)
  n119 = case shown="True" w351 {
    tunnel: w350 -> [w1026 w1399]
    tunnel: w349 -> [w1025 w1398]
    tunnel: w348 -> [w1024 w1397]
    tunnel: w347 -> [w1023 w1396]
    tunnel: w346 -> [_ w1395]
    tunnel: w345 -> [w1021 w1394]
    tunnel: w344 -> [_ w1393]
    tunnel: w343 -> [w1020 w1392]
    tunnel: w342 -> [w1022 w1387]
    tunnel: [w1026 w1336] -> w338
    tunnel: [w1025 w1337] -> w339
    tunnel: [w1024 w1335] -> w340
    tunnel: [w1023 w1334] -> w341
    tunnel: [w1022 w1085] -> w333
    tunnel: [w1020 w1333] -> w327
    tunnel: [_ w1332] -> w328
    tunnel: [w1021 w1331] -> w329
    tunnel: w295 -> [_ w1330]
    tunnel: w294 -> [w1019 w1329]
    tunnel: w293 -> [_ w1328]
    tunnel: w292 -> [w1018 w1327]
    tunnel: [w1019 w1311] -> w285
    tunnel: [w1018 w1305] -> w283
    tunnel: [_ w1295] -> w284
    tunnel: w269 -> [_ w1293]
    tunnel: w123 -> [w1017 w1291]
    tunnel: w122 -> [_ w1289]
    tunnel: w121 -> [w1016 w1287]
    tunnel: w120 -> [_ w1285]
    tunnel: w119 -> [w1015 w1283]
    tunnel: w118 -> [_ w1281]
    tunnel: w117 -> [w1014 w1279]
    tunnel: w116 -> [_ w1277]
    tunnel: w115 -> [w1013 w1275]
    tunnel: w114 -> [_ w1273]
    tunnel: w113 -> [w1012 w1271]
    tunnel: w112 -> [_ w1269]
    tunnel: w111 -> [w1011 w1267]
    tunnel: w110 -> [_ w1265]
    tunnel: w109 -> [w1010 w1263]
    tunnel: w108 -> [_ w1261]
    tunnel: w107 -> [w1009 w1259]
    tunnel: w106 -> [_ w1257]
    tunnel: w105 -> [w1008 w1255]
    tunnel: w104 -> [_ w1254]
    tunnel: w103 -> [_ w1250]
    tunnel: w102 -> [_ w1248]
    tunnel: w101 -> [_ w1246]
    tunnel: w100 -> [_ w1244]
    tunnel: w99 -> [_ w1242]
    tunnel: [w1017 w1092] -> w52
    tunnel: [_ w1091] -> w53
    tunnel: [w1016 w1090] -> w54
    tunnel: [w1015 w1081] -> w55
    tunnel: [_ w1080] -> w56
    tunnel: [w1014 w1079] -> w57
    tunnel: [w1013 w1078] -> w58
    tunnel: [_ w1077] -> w59
    tunnel: [w1012 w1076] -> w60
    tunnel: [w1011 w1075] -> w61
    tunnel: [_ w1074] -> w62
    tunnel: [w1010 w1073] -> w63
    tunnel: [w1009 w1072] -> w66
    tunnel: [_ w1071] -> w65
    tunnel: [w1008 w1070] -> w64
    tunnel: w16 -> [_ w1069]
    tunnel: w15 -> [w1007 w1068]
    tunnel: w14 -> [_ w1067]
    tunnel: w13 -> [w1006 w1066]
    tunnel: w12 -> [_ w1065]
    tunnel: [w1007 w1029] -> w5
    tunnel: [_ w1028] -> w4
    tunnel: [w1006 w1027] -> w3
    frame False {
    }
    frame True {
      n120 = flat-sequence {
        tunnel: w1399 -> [w1467]
        tunnel: w1398 -> [w1464]
        tunnel: w1397 -> [w1466]
        tunnel: w1396 -> [w1458]
        tunnel: w1395 -> [w1463]
        tunnel: w1394 -> [w1462]
        tunnel: w1393 -> [w1461]
        tunnel: w1392 -> [w1460]
        tunnel: [w1467] -> w1391
        tunnel: [w1466] -> w1390
        tunnel: [w1402] -> w1389
        tunnel: [w1465] -> w1388
        tunnel: w1387 -> [w1465]
        tunnel: [w1401] -> w1386
        tunnel: [w1463] -> w1385
        tunnel: [w1462] -> w1384
        tunnel: [w1461] -> w1383
        tunnel: [w1460] -> w1382
        tunnel: [w1459] -> w1381
        tunnel: w1330 -> [w1455]
        tunnel: w1329 -> [w1454]
        tunnel: w1328 -> [w1457]
        tunnel: w1327 -> [w1456]
        tunnel: [w1455] -> w1322
        tunnel: [w1457] -> w1317
        tunnel: [w1454] -> w1316
        tunnel: [w1456] -> w1310
        tunnel: [w1453] -> w1304
        tunnel: [w1426] -> w1294
        tunnel: w1293 -> [w1426]
        tunnel: [w1425] -> w1292
        tunnel: w1291 -> [w1425]
        tunnel: [w1450] -> w1290
        tunnel: w1289 -> [w1450]
        tunnel: [w1449] -> w1288
        tunnel: w1287 -> [w1449]
        tunnel: [w1422] -> w1286
        tunnel: w1285 -> [w1422]
        tunnel: [w1421] -> w1284
        tunnel: w1283 -> [w1421]
        tunnel: [w1424] -> w1282
        tunnel: w1281 -> [w1424]
        tunnel: [w1423] -> w1280
        tunnel: w1279 -> [w1423]
        tunnel: [w1420] -> w1278
        tunnel: w1277 -> [w1420]
        tunnel: [w1419] -> w1276
        tunnel: w1275 -> [w1419]
        tunnel: [w1448] -> w1274
        tunnel: w1273 -> [w1448]
        tunnel: [w1447] -> w1272
        tunnel: w1271 -> [w1447]
        tunnel: [w1418] -> w1270
        tunnel: w1269 -> [w1418]
        tunnel: [w1417] -> w1268
        tunnel: w1267 -> [w1417]
        tunnel: [w1446] -> w1266
        tunnel: w1265 -> [w1446]
        tunnel: [w1445] -> w1264
        tunnel: w1263 -> [w1445]
        tunnel: [w1416] -> w1262
        tunnel: w1261 -> [w1416]
        tunnel: [w1415] -> w1260
        tunnel: w1259 -> [w1415]
        tunnel: [w1444] -> w1258
        tunnel: w1257 -> [w1444]
        tunnel: [w1443] -> w1256
        tunnel: w1255 -> [w1443]
        tunnel: w1254 -> [w1442]
        tunnel: [w1442] -> w1253
        tunnel: [w1441] -> w1251
        tunnel: w1250 -> [w1441]
        tunnel: [w1440] -> w1249
        tunnel: w1248 -> [w1440]
        tunnel: [w1439] -> w1247
        tunnel: w1246 -> [w1439]
        tunnel: [w1438] -> w1245
        tunnel: w1244 -> [w1438]
        tunnel: [w1437] -> w1243
        tunnel: w1242 -> [w1437]
        tunnel: [w1414] -> w1241
        tunnel: [w1413] -> w1240
        tunnel: [w1412] -> w1239
        tunnel: [w1411] -> w1238
        tunnel: [w1410] -> w1237
        tunnel: w1069 -> [w1405]
        tunnel: w1068 -> [w1406]
        tunnel: w1067 -> [w1409]
        tunnel: w1066 -> [w1408]
        tunnel: w1065 -> [w1407]
        tunnel: [w1405] -> w1060
        tunnel: [w1406] -> w1055
        tunnel: [w1409] -> w1050
        tunnel: [w1408] -> w1046
        tunnel: [w1407] -> w1041
        tunnel: [w1400] -> w1040
        tunnel: w1391 -> [w1615]
        tunnel: w1390 -> [w1618]
        tunnel: w1389 -> [w1617]
        tunnel: w1388 -> [w1603]
        tunnel: w1386 -> [w1616]
        tunnel: w1385 -> [w1619]
        tunnel: w1384 -> [w1620]
        tunnel: w1383 -> [w1622]
        tunnel: w1382 -> [w1621]
        tunnel: w1381 -> [w1598]
        tunnel: [w1622] -> w1380
        tunnel: [w1621] -> w1379
        tunnel: [w1620] -> w1378
        tunnel: [w1619] -> w1377
        tunnel: [w1618] -> w1376
        tunnel: [w1617] -> w1375
        tunnel: [w1616] -> w1374
        tunnel: [w1615] -> w1373
        tunnel: [w1602] -> w1372
        tunnel: [w1600] -> w1371
        tunnel: [w1614] -> w1323
        tunnel: w1322 -> [w1614]
        tunnel: [w1613] -> w1318
        tunnel: w1317 -> [w1613]
        tunnel: w1316 -> [w1612]
        tunnel: [w1612] -> w1315
        tunnel: w1310 -> [w1611]
        tunnel: [w1611] -> w1309
        tunnel: w1304 -> [w1597]
        tunnel: [w1601] -> w1303
        tunnel: [w1599] -> w1302
        tunnel: w1294 -> [w1591]
        tunnel: w1292 -> [w1590]
        tunnel: w1290 -> [w1589]
        tunnel: w1288 -> [w1588]
        tunnel: w1286 -> [w1586]
        tunnel: w1284 -> [w1585]
        tunnel: w1282 -> [w1584]
        tunnel: w1280 -> [w1583]
        tunnel: w1278 -> [w1581]
        tunnel: w1276 -> [w1580]
        tunnel: w1274 -> [w1579]
        tunnel: w1272 -> [w1578]
        tunnel: w1270 -> [w1576]
        tunnel: w1268 -> [w1575]
        tunnel: w1266 -> [w1574]
        tunnel: w1264 -> [w1573]
        tunnel: w1262 -> [w1571]
        tunnel: w1260 -> [w1570]
        tunnel: w1258 -> [w1569]
        tunnel: w1256 -> [w1568]
        tunnel: w1253 -> [w1610]
        tunnel: [w1610] -> w1252
        tunnel: w1251 -> [w1587]
        tunnel: w1249 -> [w1582]
        tunnel: w1247 -> [w1577]
        tunnel: w1245 -> [w1572]
        tunnel: w1243 -> [w1567]
        tunnel: w1241 -> [w1596]
        tunnel: w1240 -> [w1595]
        tunnel: w1239 -> [w1594]
        tunnel: w1238 -> [w1593]
        tunnel: w1237 -> [w1592]
        tunnel: [w1549] -> w1236
        tunnel: [w1591] -> w1232
        tunnel: [w1590] -> w1228
        tunnel: [w1589] -> w1224
        tunnel: [w1588] -> w1220
        tunnel: [w1587] -> w1216
        tunnel: [w1586] -> w1212
        tunnel: [w1585] -> w1208
        tunnel: [w1584] -> w1204
        tunnel: [w1583] -> w1201
        tunnel: [w1582] -> w1197
        tunnel: [w1581] -> w1193
        tunnel: [w1580] -> w1189
        tunnel: [w1579] -> w1185
        tunnel: [w1578] -> w1181
        tunnel: [w1577] -> w1178
        tunnel: [w1576] -> w1174
        tunnel: [w1575] -> w1170
        tunnel: [w1574] -> w1166
        tunnel: [w1573] -> w1163
        tunnel: [w1572] -> w1159
        tunnel: [w1571] -> w1155
        tunnel: [w1570] -> w1151
        tunnel: [w1569] -> w1147
        tunnel: [w1568] -> w1144
        tunnel: [w1567] -> w1140
        tunnel: [w1566] -> w1132
        tunnel: [w1565] -> w1130
        tunnel: [w1564] -> w1128
        tunnel: [w1563] -> w1126
        tunnel: [w1562] -> w1124
        tunnel: [w1561] -> w1122
        tunnel: [w1560] -> w1120
        tunnel: [w1559] -> w1118
        tunnel: [w1558] -> w1116
        tunnel: [w1557] -> w1114
        tunnel: [w1556] -> w1061
        tunnel: w1060 -> [w1556]
        tunnel: [w1555] -> w1056
        tunnel: w1055 -> [w1555]
        tunnel: [w1554] -> w1051
        tunnel: w1050 -> [w1554]
        tunnel: [w1553] -> w1047
        tunnel: w1046 -> [w1553]
        tunnel: [w1552] -> w1042
        tunnel: w1041 -> [w1552]
        tunnel: w1040 -> [w1551]
        tunnel: [w1551] -> w1036
        tunnel: [w1548] -> w1035
        tunnel: w1380 -> [w1695]
        tunnel: w1379 -> [w1696]
        tunnel: w1378 -> [w1706]
        tunnel: w1377 -> [w1705]
        tunnel: w1376 -> [w1704]
        tunnel: w1375 -> [w1703]
        tunnel: w1374 -> [w1702]
        tunnel: w1373 -> [w1701]
        tunnel: w1372 -> [w1700]
        tunnel: w1371 -> [w1699]
        tunnel: [w1698] -> w1370
        tunnel: [w1697] -> w1369
        tunnel: [w1706] -> w1368
        tunnel: [w1705] -> w1367
        tunnel: [w1704] -> w1366
        tunnel: [w1703] -> w1365
        tunnel: [w1702] -> w1364
        tunnel: [w1701] -> w1363
        tunnel: [w1700] -> w1362
        tunnel: [w1699] -> w1361
        tunnel: [w1675] -> w1360
        tunnel: [w1693] -> w1324
        tunnel: w1323 -> [w1693]
        tunnel: [w1687] -> w1319
        tunnel: w1318 -> [w1689]
        tunnel: w1315 -> [w1692]
        tunnel: [w1692] -> w1314
        tunnel: w1309 -> [w1688]
        tunnel: [w1686] -> w1308
        tunnel: w1303 -> [w1691]
        tunnel: w1302 -> [w1690]
        tunnel: [w1691] -> w1299
        tunnel: [w1690] -> w1296
        tunnel: w1252 -> [w1674]
        tunnel: w1236 -> [w1694]
        tunnel: [w1685] -> w1233
        tunnel: w1232 -> [w1685]
        tunnel: [w1684] -> w1229
        tunnel: w1228 -> [w1684]
        tunnel: [w1667] -> w1225
        tunnel: w1224 -> [w1672]
        tunnel: [w1668] -> w1221
        tunnel: w1220 -> [w1671]
        tunnel: [w1669] -> w1217
        tunnel: w1216 -> [w1670]
        tunnel: [w1683] -> w1213
        tunnel: w1212 -> [w1683]
        tunnel: [w1682] -> w1209
        tunnel: w1208 -> [w1682]
        tunnel: [w1661] -> w1205
        tunnel: w1204 -> [w1666]
        tunnel: w1201 -> [w1665]
        tunnel: [w1663] -> w1198
        tunnel: w1197 -> [w1664]
        tunnel: [w1681] -> w1194
        tunnel: w1193 -> [w1681]
        tunnel: [w1680] -> w1190
        tunnel: w1189 -> [w1680]
        tunnel: [w1657] -> w1186
        tunnel: w1185 -> [w1658]
        tunnel: [w1656] -> w1182
        tunnel: w1181 -> [w1659]
        tunnel: w1178 -> [w1660]
        tunnel: [w1679] -> w1175
        tunnel: w1174 -> [w1679]
        tunnel: [w1678] -> w1171
        tunnel: w1170 -> [w1678]
        tunnel: [w1649] -> w1167
        tunnel: w1166 -> [w1654]
        tunnel: w1163 -> [w1653]
        tunnel: [w1651] -> w1160
        tunnel: w1159 -> [w1652]
        tunnel: [w1677] -> w1156
        tunnel: w1155 -> [w1677]
        tunnel: [w1676] -> w1152
        tunnel: w1151 -> [w1676]
        tunnel: [w1643] -> w1148
        tunnel: w1147 -> [w1648]
        tunnel: w1144 -> [w1647]
        tunnel: [w1645] -> w1141
        tunnel: w1140 -> [w1646]
        tunnel: [w1673] -> w1139
        tunnel: [w1662] -> w1137
        tunnel: [w1655] -> w1136
        tunnel: [w1650] -> w1135
        tunnel: [w1644] -> w1134
        tunnel: [w1642] -> w1133
        tunnel: w1132 -> [w1642]
        tunnel: [w1641] -> w1131
        tunnel: w1130 -> [w1641]
        tunnel: [w1640] -> w1129
        tunnel: w1128 -> [w1640]
        tunnel: [w1639] -> w1127
        tunnel: w1126 -> [w1639]
        tunnel: [w1638] -> w1125
        tunnel: w1124 -> [w1638]
        tunnel: [w1637] -> w1123
        tunnel: w1122 -> [w1637]
        tunnel: [w1636] -> w1121
        tunnel: w1120 -> [w1636]
        tunnel: [w1635] -> w1119
        tunnel: w1118 -> [w1635]
        tunnel: [w1634] -> w1117
        tunnel: w1116 -> [w1634]
        tunnel: [w1633] -> w1115
        tunnel: w1114 -> [w1633]
        tunnel: [w1632] -> w1062
        tunnel: w1061 -> [w1632]
        tunnel: [w1631] -> w1057
        tunnel: w1056 -> [w1631]
        tunnel: [w1625] -> w1052
        tunnel: w1051 -> [w1628]
        tunnel: w1047 -> [w1627]
        tunnel: [w1623] -> w1043
        tunnel: w1042 -> [w1626]
        tunnel: [w1630] -> w1037
        tunnel: w1036 -> [w1630]
        tunnel: w1035 -> [w1629]
        tunnel: [w1629] -> w1032
        tunnel: [w1624] -> w1031
        tunnel: w1370 -> [w1853]
        tunnel: w1369 -> [w1855]
        tunnel: w1368 -> [w1849]
        tunnel: w1367 -> [w1852]
        tunnel: w1366 -> [w1862]
        tunnel: w1365 -> [w1861]
        tunnel: w1364 -> [w1860]
        tunnel: w1363 -> [w1859]
        tunnel: w1362 -> [w1858]
        tunnel: w1361 -> [w1857]
        tunnel: w1360 -> [w1851]
        tunnel: [w1853] -> w1359
        tunnel: [w1855] -> w1358
        tunnel: [w1850] -> w1357
        tunnel: [w1852] -> w1356
        tunnel: [w1862] -> w1355
        tunnel: [w1861] -> w1354
        tunnel: [w1860] -> w1353
        tunnel: [w1859] -> w1352
        tunnel: [w1858] -> w1351
        tunnel: [w1857] -> w1350
        tunnel: [w1839] -> w1349
        tunnel: [w1843] -> w1325
        tunnel: w1324 -> [w1843]
        tunnel: [w1844] -> w1320
        tunnel: w1319 -> [w1844]
        tunnel: w1314 -> [w1841]
        tunnel: [w1840] -> w1313
        tunnel: w1308 -> [w1845]
        tunnel: [w1845] -> w1306
        tunnel: [w1848] -> w1300
        tunnel: w1299 -> [w1848]
        tunnel: [w1847] -> w1297
        tunnel: w1296 -> [w1847]
        tunnel: [w1805] -> w1234
        tunnel: w1233 -> [w1805]
        tunnel: [w1813] -> w1230
        tunnel: w1229 -> [w1817]
        tunnel: [w1808] -> w1226
        tunnel: w1225 -> [w1808]
        tunnel: [w1816] -> w1222
        tunnel: w1221 -> [w1816]
        tunnel: [w1809] -> w1218
        tunnel: w1217 -> [w1810]
        tunnel: [w1806] -> w1214
        tunnel: w1213 -> [w1806]
        tunnel: [w1812] -> w1210
        tunnel: w1209 -> [w1815]
        tunnel: [w1807] -> w1206
        tunnel: w1205 -> [w1807]
        tunnel: [w1814] -> w1202
        tunnel: [w1803] -> w1199
        tunnel: w1198 -> [w1804]
        tunnel: [w1789] -> w1195
        tunnel: w1194 -> [w1789]
        tunnel: [w1786] -> w1191
        tunnel: w1190 -> [w1802]
        tunnel: [w1790] -> w1187
        tunnel: w1186 -> [w1790]
        tunnel: [w1801] -> w1183
        tunnel: w1182 -> [w1801]
        tunnel: [w1787] -> w1179
        tunnel: [w1792] -> w1176
        tunnel: w1175 -> [w1792]
        tunnel: [w1784] -> w1172
        tunnel: w1171 -> [w1800]
        tunnel: [w1793] -> w1168
        tunnel: w1167 -> [w1793]
        tunnel: [w1799] -> w1164
        tunnel: [w1785] -> w1161
        tunnel: w1160 -> [w1791]
        tunnel: [w1795] -> w1157
        tunnel: w1156 -> [w1795]
        tunnel: [w1782] -> w1153
        tunnel: w1152 -> [w1798]
        tunnel: [w1796] -> w1149
        tunnel: w1148 -> [w1796]
        tunnel: [w1797] -> w1145
        tunnel: [w1783] -> w1142
        tunnel: w1141 -> [w1794]
        tunnel: w1139 -> [w1838]
        tunnel: [w1837] -> w1138
        tunnel: w1137 -> [w1814]
        tunnel: w1136 -> [w1788]
        tunnel: w1135 -> [w1799]
        tunnel: w1134 -> [w1797]
        tunnel: w1133 -> [w1828]
        tunnel: w1131 -> [w1811]
        tunnel: w1129 -> [w1829]
        tunnel: w1127 -> [w1830]
        tunnel: w1125 -> [w1831]
        tunnel: w1123 -> [w1832]
        tunnel: w1121 -> [w1833]
        tunnel: w1119 -> [w1834]
        tunnel: w1117 -> [w1835]
        tunnel: w1115 -> [w1836]
        tunnel: [w1836] -> w1112
        tunnel: [w1835] -> w1110
        tunnel: [w1834] -> w1108
        tunnel: [w1833] -> w1106
        tunnel: [w1832] -> w1104
        tunnel: [w1831] -> w1102
        tunnel: [w1830] -> w1100
        tunnel: [w1829] -> w1098
        tunnel: [w1811] -> w1096
        tunnel: [w1828] -> w1094
        tunnel: [w1771] -> w1063
        tunnel: w1062 -> [w1771]
        tunnel: [w1774] -> w1058
        tunnel: w1057 -> [w1775]
        tunnel: [w1772] -> w1053
        tunnel: w1052 -> [w1772]
        tunnel: [w1778] -> w1048
        tunnel: [w1776] -> w1044
        tunnel: w1043 -> [w1777]
        tunnel: [w1781] -> w1038
        tunnel: w1037 -> [w1781]
        tunnel: [w1780] -> w1033
        tunnel: w1032 -> [w1780]
        tunnel: w1031 -> [w1778]
        tunnel: w1359 -> [w2026]
        tunnel: w1358 -> [w2025]
        tunnel: w1357 -> [w2015]
        tunnel: w1356 -> [w2021]
        tunnel: w1355 -> [w2024]
        tunnel: w1354 -> [w2020]
        tunnel: w1353 -> [w2019]
        tunnel: w1352 -> [w2023]
        tunnel: w1351 -> [w2018]
        tunnel: w1350 -> [w2014]
        tunnel: w1349 -> [w2022]
        tunnel: [w2026] -> w1348
        tunnel: [w2025] -> w1347
        tunnel: [w2015] -> w1346
        tunnel: [w2021] -> w1345
        tunnel: [w2024] -> w1344
        tunnel: [w1928] -> w1343
        tunnel: [w1927] -> w1342
        tunnel: [w2023] -> w1341
        tunnel: [w2017] -> w1340
        tunnel: [w2014] -> w1339
        tunnel: [w2022] -> w1338
        tunnel: [w2006] -> w1326
        tunnel: w1325 -> [w2006]
        tunnel: [w2012] -> w1321
        tunnel: w1320 -> [w2012]
        tunnel: w1313 -> [w2008]
        tunnel: [w2008] -> w1312
        tunnel: [w2011] -> w1307
        tunnel: w1306 -> [w2011]
        tunnel: [w2002] -> w1301
        tunnel: w1300 -> [w2003]
        tunnel: [w2009] -> w1298
        tunnel: w1297 -> [w2009]
        tunnel: [w1965] -> w1235
        tunnel: w1234 -> [w1965]
        tunnel: [w1979] -> w1231
        tunnel: w1230 -> [w1979]
        tunnel: [w2001] -> w1227
        tunnel: w1226 -> [w2001]
        tunnel: [w2000] -> w1223
        tunnel: w1222 -> [w2000]
        tunnel: [w1999] -> w1219
        tunnel: w1218 -> [w1999]
        tunnel: [w1964] -> w1215
        tunnel: w1214 -> [w1964]
        tunnel: [w1976] -> w1211
        tunnel: w1210 -> [w1976]
        tunnel: [w1998] -> w1207
        tunnel: w1206 -> [w1998]
        tunnel: [w1997] -> w1203
        tunnel: w1202 -> [w1997]
        tunnel: [w1996] -> w1200
        tunnel: w1199 -> [w1996]
        tunnel: [w1960] -> w1196
        tunnel: w1195 -> [w1960]
        tunnel: [w1974] -> w1192
        tunnel: w1191 -> [w1974]
        tunnel: [w1995] -> w1188
        tunnel: w1187 -> [w1995]
        tunnel: [w1994] -> w1184
        tunnel: w1183 -> [w1994]
        tunnel: [w1993] -> w1180
        tunnel: w1179 -> [w1993]
        tunnel: [w1959] -> w1177
        tunnel: w1176 -> [w1959]
        tunnel: [w1972] -> w1173
        tunnel: w1172 -> [w1972]
        tunnel: [w1992] -> w1169
        tunnel: w1168 -> [w1992]
        tunnel: [w1991] -> w1165
        tunnel: w1164 -> [w1991]
        tunnel: [w1990] -> w1162
        tunnel: w1161 -> [w1990]
        tunnel: [w1957] -> w1158
        tunnel: w1157 -> [w1957]
        tunnel: [w1970] -> w1154
        tunnel: w1153 -> [w1970]
        tunnel: [w1989] -> w1150
        tunnel: w1149 -> [w1989]
        tunnel: [w1988] -> w1146
        tunnel: w1145 -> [w1988]
        tunnel: [w1987] -> w1143
        tunnel: w1142 -> [w1987]
        tunnel: w1138 -> [w1986]
        tunnel: [w1941] -> w1113
        tunnel: w1112 -> [w1956]
        tunnel: [w1971] -> w1111
        tunnel: w1110 -> [w1971]
        tunnel: [w1942] -> w1109
        tunnel: w1108 -> [w1958]
        tunnel: [w1973] -> w1107
        tunnel: w1106 -> [w1973]
        tunnel: [w1943] -> w1105
        tunnel: w1104 -> [w1961]
        tunnel: [w1975] -> w1103
        tunnel: w1102 -> [w1975]
        tunnel: [w1944] -> w1101
        tunnel: w1100 -> [w1962]
        tunnel: [w1977] -> w1099
        tunnel: w1098 -> [w1977]
        tunnel: [w1945] -> w1097
        tunnel: w1096 -> [w1963]
        tunnel: [w1980] -> w1095
        tunnel: w1094 -> [w1980]
        tunnel: [w1986] -> w1093
        tunnel: [w1933] -> w1064
        tunnel: w1063 -> [w1933]
        tunnel: [w1934] -> w1059
        tunnel: w1058 -> [w1934]
        tunnel: [w1940] -> w1054
        tunnel: w1053 -> [w1940]
        tunnel: [w1939] -> w1049
        tunnel: w1048 -> [w1939]
        tunnel: [w1938] -> w1045
        tunnel: w1044 -> [w1938]
        tunnel: [w1929] -> w1039
        tunnel: w1038 -> [w1930]
        tunnel: [w1935] -> w1034
        tunnel: w1033 -> [w1935]
        tunnel: w1348 -> [w2198]
        tunnel: w1347 -> [w2197]
        tunnel: w1346 -> [w2196]
        tunnel: w1345 -> [w2195]
        tunnel: w1344 -> [w2194]
        tunnel: w1343 -> [w2193]
        tunnel: w1342 -> [w2192]
        tunnel: w1341 -> [w2191]
        tunnel: w1340 -> [w2189]
        tunnel: w1339 -> [w2187]
        tunnel: w1338 -> [w2186]
        tunnel: [w2198] -> _
        tunnel: [w2197] -> w1333
        tunnel: [w2196] -> w1331
        tunnel: [w2195] -> _
        tunnel: [w2194] -> w1335
        tunnel: [w2193] -> w1334
        tunnel: [w2192] -> w1337
        tunnel: [w2191] -> w1336
        tunnel: [w2189] -> _
        tunnel: [w2188] -> w1332
        tunnel: [w2157] -> w1086
        tunnel: [w2185] -> _
        tunnel: w1326 -> [w2185]
        tunnel: [w2184] -> _
        tunnel: w1321 -> [w2184]
        tunnel: w1312 -> [w2183]
        tunnel: [w2183] -> w1311
        tunnel: [w2182] -> w1305
        tunnel: w1307 -> [w2182]
        tunnel: [w2179] -> _
        tunnel: w1301 -> [w2179]
        tunnel: [w2178] -> w1295
        tunnel: w1298 -> [w2180]
        tunnel: [w2177] -> _
        tunnel: w1235 -> [w2177]
        tunnel: [w2176] -> w1092
        tunnel: w1231 -> [w2176]
        tunnel: [w2175] -> _
        tunnel: w1227 -> [w2175]
        tunnel: [w2174] -> w1090
        tunnel: w1223 -> [w2174]
        tunnel: [w2133] -> w1089
        tunnel: w1219 -> [w2135]
        tunnel: [w2173] -> _
        tunnel: w1215 -> [w2173]
        tunnel: [w2172] -> w1081
        tunnel: w1211 -> [w2172]
        tunnel: [w2171] -> _
        tunnel: w1207 -> [w2171]
        tunnel: [w2170] -> w1079
        tunnel: w1203 -> [w2170]
        tunnel: [w2131] -> w1088
        tunnel: w1200 -> [w2136]
        tunnel: [w2169] -> _
        tunnel: w1196 -> [w2169]
        tunnel: [w2168] -> w1078
        tunnel: w1192 -> [w2168]
        tunnel: [w2167] -> _
        tunnel: w1188 -> [w2167]
        tunnel: [w2166] -> w1076
        tunnel: w1184 -> [w2166]
        tunnel: [w2129] -> w1084
        tunnel: w1180 -> [w2137]
        tunnel: [w2165] -> _
        tunnel: w1177 -> [w2165]
        tunnel: [w2164] -> w1075
        tunnel: w1173 -> [w2164]
        tunnel: [w2163] -> _
        tunnel: w1169 -> [w2163]
        tunnel: [w2162] -> w1073
        tunnel: w1165 -> [w2162]
        tunnel: [w2127] -> w1083
        tunnel: w1162 -> [w2138]
        tunnel: [w2161] -> _
        tunnel: w1158 -> [w2161]
        tunnel: [w2160] -> w1072
        tunnel: w1154 -> [w2160]
        tunnel: [w2159] -> _
        tunnel: w1150 -> [w2159]
        tunnel: [w2158] -> w1070
        tunnel: w1146 -> [w2158]
        tunnel: [w2125] -> w1082
        tunnel: w1143 -> [w2139]
        tunnel: [w2140] -> _
        tunnel: w1113 -> [w2140]
        tunnel: [w2126] -> w1071
        tunnel: w1111 -> [w2145]
        tunnel: [w2141] -> _
        tunnel: w1109 -> [w2141]
        tunnel: [w2128] -> w1074
        tunnel: w1107 -> [w2146]
        tunnel: [w2142] -> _
        tunnel: w1105 -> [w2142]
        tunnel: [w2130] -> w1077
        tunnel: w1103 -> [w2147]
        tunnel: [w2143] -> _
        tunnel: w1101 -> [w2143]
        tunnel: [w2132] -> w1080
        tunnel: w1099 -> [w2148]
        tunnel: [w2144] -> _
        tunnel: w1097 -> [w2144]
        tunnel: [w2134] -> w1091
        tunnel: w1095 -> [w2149]
        tunnel: w1093 -> [w2156]
        tunnel: [w2155] -> w1087
        tunnel: w1064 -> [w2124]
        tunnel: w1059 -> [w2123]
        tunnel: w1054 -> [w2122]
        tunnel: w1049 -> [w2121]
        tunnel: w1045 -> [w2116]
        tunnel: w1039 -> [w2119]
        tunnel: [w2124] -> _
        tunnel: [w2123] -> w1029
        tunnel: [w2119] -> _
        tunnel: [w2122] -> _
        tunnel: [w2121] -> w1027
        tunnel: [w2115] -> w1030
        tunnel: w1034 -> [w2118]
        tunnel: [w2117] -> w1028
        frame #0 {
          # "Use Excel\nto add\nheaders"
          n121 = case shown="True" w1462 {
            selector: w1462 -> [_ w1546]
            tunnel: w1463 -> [_ w1545]
            tunnel: w1458 -> [w1539 w1544]
            tunnel: w1464 -> [w1538 w1543]
            tunnel: [w1538 w1541] -> w1451
            tunnel: [w1539 w1542] -> w1452
            tunnel: [_ w1540] -> w1459
            frame False {
            }
            frame True {
              n122 = call "myRIO_BRig_Host_formatData_getHeaders_dataBlock.vi"() -> ("output_stringArray_dataBlock"=w1547:string[])  [unwired: 11 in]
              n123 = call "myRIO_BRig_Host_formatData_test3_p2.vi"("input_headers"=w1547, "input_error"=w1543, "input_Iexist"=w1546, "input_filePath"=w1545, "input_hdl_Workbooks"=w1544) -> ("output_error"=w1541:errorcluster, "output_newFilePath"=w1540:path, "output_hdl_Worksbooks"=w1542:refnum<k7>)  [unwired: 4 in]
            }
          }
          n124 = case shown="True" w1454 {
            selector: w1454 -> [_ w1536]
            tunnel: w1455 -> [_ w1535]
            tunnel: w1452 -> [w1529 w1534]
            tunnel: w1451 -> [w1528 w1533]
            tunnel: [w1528 w1531] -> w1435
            tunnel: [w1529 w1532] -> w1436
            tunnel: [_ w1530] -> w1453
            frame False {
            }
            frame True {
              n125 = call "myRIO_BRig_Host_formatData_getHeaders_dataCurrent.vi"() -> ("output_stringArray_dataCurrent"=w1537:string[])  [unwired: 11 in]
              n126 = call "myRIO_BRig_Host_formatData_test3_p2.vi"("input_headers"=w1537, "input_error"=w1533, "input_Iexist"=w1536, "input_filePath"=w1535, "input_hdl_Workbooks"=w1534) -> ("output_error"=w1531:errorcluster, "output_newFilePath"=w1530:path, "output_hdl_Worksbooks"=w1532:refnum<k7>)  [unwired: 4 in]
            }
          }
          n127 = case shown="True" w1425 {
            selector: w1425 -> [_ w1526]
            tunnel: w1426 -> [_ w1525]
            tunnel: w1436 -> [w1519 w1524]
            tunnel: w1435 -> [w1518 w1523]
            tunnel: [w1518 w1521] -> w1433
            tunnel: [w1519 w1522] -> w1434
            tunnel: [_ w1520] -> w1414
            frame False {
            }
            frame True {
              n128 = call "myRIO_BRig_Host_formatData_getHeaders_dataExp.vi"() -> ("output_stringArray_dataExp"=w1527:string[])  [unwired: 11 in]
              n129 = call "myRIO_BRig_Host_formatData_test3_p2.vi"("input_headers"=w1527, "input_error"=w1523, "input_Iexist"=w1526, "input_filePath"=w1525, "input_hdl_Workbooks"=w1524) -> ("output_error"=w1521:errorcluster, "output_newFilePath"=w1520:path, "output_hdl_Worksbooks"=w1522:refnum<k7>)  [unwired: 4 in]
            }
          }
          n130 = case shown="True" w1421 {
            selector: w1421 -> [_ w1516]
            tunnel: w1422 -> [_ w1515]
            tunnel: w1434 -> [w1509 w1514]
            tunnel: w1433 -> [w1508 w1513]
            tunnel: [w1508 w1511] -> w1431
            tunnel: [w1509 w1512] -> w1432
            tunnel: [_ w1510] -> w1413
            frame False {
            }
            frame True {
              n131 = call "myRIO_BRig_Host_formatData_getHeaders_dataLC.vi"() -> ("output_stringArray_dataLC"=w1517:string[])  [unwired: 11 in]
              n132 = call "myRIO_BRig_Host_formatData_test3_p2.vi"("input_headers"=w1517, "input_error"=w1513, "input_Iexist"=w1516, "input_filePath"=w1515, "input_hdl_Workbooks"=w1514) -> ("output_error"=w1511:errorcluster, "output_newFilePath"=w1510:path, "output_hdl_Worksbooks"=w1512:refnum<k7>)  [unwired: 4 in]
            }
          }
          n133 = case shown="True" w1419 {
            selector: w1419 -> [_ w1506]
            tunnel: w1420 -> [_ w1505]
            tunnel: w1432 -> [w1499 w1504]
            tunnel: w1431 -> [w1498 w1503]
            tunnel: [w1498 w1501] -> w1429
            tunnel: [w1499 w1502] -> w1430
            tunnel: [_ w1500] -> w1412
            frame False {
            }
            frame True {
              n134 = call "myRIO_BRig_Host_formatData_getHeaders_dataLick.vi"() -> ("output_stringArray_dataLick"=w1507:string[])  [unwired: 11 in]
              n135 = call "myRIO_BRig_Host_formatData_test3_p2.vi"("input_headers"=w1507, "input_error"=w1503, "input_Iexist"=w1506, "input_filePath"=w1505, "input_hdl_Workbooks"=w1504) -> ("output_error"=w1501:errorcluster, "output_newFilePath"=w1500:path, "output_hdl_Worksbooks"=w1502:refnum<k7>)  [unwired: 4 in]
            }
          }
          n136 = case shown="True" w1417 {
            selector: w1417 -> [_ w1496]
            tunnel: w1418 -> [_ w1495]
            tunnel: w1430 -> [w1489 w1494]
            tunnel: w1429 -> [w1488 w1493]
            tunnel: [w1488 w1491] -> w1427
            tunnel: [w1489 w1492] -> w1428
            tunnel: [_ w1490] -> w1411
            frame False {
            }
            frame True {
              n137 = call "myRIO_BRig_Host_formatData_getHeaders_dataMTrig.vi"() -> ("output_stringArray_dataMTrig"=w1497:string[])  [unwired: 11 in]
              n138 = call "myRIO_BRig_Host_formatData_test3_p2.vi"("input_headers"=w1497, "input_error"=w1493, "input_Iexist"=w1496, "input_filePath"=w1495, "input_hdl_Workbooks"=w1494) -> ("output_error"=w1491:errorcluster, "output_newFilePath"=w1490:path, "output_hdl_Worksbooks"=w1492:refnum<k7>)  [unwired: 4 in]
            }
          }
          n139 = case shown="True" w1415 {
            selector: w1415 -> [_ w1486]
            tunnel: w1416 -> [_ w1485]
            tunnel: w1428 -> [w1479 w1484]
            tunnel: w1427 -> [w1478 w1483]
            tunnel: [w1478 w1481] -> w1404
            tunnel: [w1479 w1482] -> w1403
            tunnel: [_ w1480] -> w1410
            frame False {
            }
            frame True {
              n140 = call "myRIO_BRig_Host_formatData_getHeaders_dataTrial.vi"() -> ("output_stringArray_dataTrial"=w1487:string[])  [unwired: 11 in]
              n141 = call "myRIO_BRig_Host_formatData_test3_p2.vi"("input_headers"=w1487, "input_error"=w1483, "input_Iexist"=w1486, "input_filePath"=w1485, "input_hdl_Workbooks"=w1484) -> ("output_error"=w1481:errorcluster, "output_newFilePath"=w1480:path, "output_hdl_Worksbooks"=w1482:refnum<k7>)  [unwired: 4 in]
            }
          }
          n142 = case shown="True" w1406 {
            selector: w1406 -> [_ w1476]
            tunnel: w1405 -> [_ w1475]
            tunnel: w1403 -> [w1469 w1474]
            tunnel: w1404 -> [w1468 w1473]
            tunnel: [w1468 w1471] -> w1401
            tunnel: [w1469 w1472] -> w1402
            tunnel: [_ w1470] -> w1400
            frame False {
            }
            frame True {
              n143 = call "myRIO_BRig_Host_formatData_getHeaders_dataAnalog.vi"() -> ("output_stringArray_dataAnalog"=w1477:string[])  [unwired: 11 in]
              n144 = call "myRIO_BRig_Host_formatData_test3_p2.vi"("input_headers"=w1477, "input_error"=w1473, "input_Iexist"=w1476, "input_filePath"=w1475, "input_hdl_Workbooks"=w1474) -> ("output_error"=w1471:errorcluster, "output_newFilePath"=w1470:path, "output_hdl_Worksbooks"=w1472:refnum<k7>)  [unwired: 4 in]
            }
          }
        }
        frame #1 {
          # "Check if\nfile was\ncreated"
          n145 = call "myRIO_BRig_generic_pathExists_fast_pathInput.vi"("input_error"=w1603, "input_filePath"=w1598) -> ("output_error"=w1609:errorcluster, "output_Iexist"=w1600:bool, "output_filePath"=w1602:path)  [unwired: 7 in]
          n146 = call "myRIO_BRig_generic_pathExists_fast_pathInput.vi"("input_error"=w1609, "input_filePath"=w1597) -> ("output_error"=w1608:errorcluster, "output_Iexist"=w1599:bool, "output_filePath"=w1601:path)  [unwired: 7 in]
          n147 = call "myRIO_BRig_generic_pathExists_fast_pathInput.vi"("input_error"=w1608, "input_filePath"=w1596) -> ("output_error"=w1607:errorcluster, "output_Iexist"=w1566:bool, "output_filePath"=w1565:path)  [unwired: 7 in]
          n148 = call "myRIO_BRig_generic_pathExists_fast_pathInput.vi"("input_error"=w1607, "input_filePath"=w1595) -> ("output_error"=w1606:errorcluster, "output_Iexist"=w1564:bool, "output_filePath"=w1563:path)  [unwired: 7 in]
          n149 = call "myRIO_BRig_generic_pathExists_fast_pathInput.vi"("input_error"=w1606, "input_filePath"=w1594) -> ("output_error"=w1605:errorcluster, "output_Iexist"=w1562:bool, "output_filePath"=w1561:path)  [unwired: 7 in]
          n150 = call "myRIO_BRig_generic_pathExists_fast_pathInput.vi"("input_error"=w1605, "input_filePath"=w1593) -> ("output_error"=w1604:errorcluster, "output_Iexist"=w1560:bool, "output_filePath"=w1559:path)  [unwired: 7 in]
          n151 = call "myRIO_BRig_generic_pathExists_fast_pathInput.vi"("input_error"=w1604, "input_filePath"=w1592) -> ("output_error"=w1550:errorcluster, "output_Iexist"=w1558:bool, "output_filePath"=w1557:path)  [unwired: 7 in]
          n152 = call "myRIO_BRig_generic_pathExists_fast_pathInput.vi"("input_error"=w1550) -> ("output_error"=w1549:errorcluster, "output_Iexist"=w1548:bool)  [unwired: 8 in, 1 out]
        }
        frame #2 {
          # "Re-check\noriginal files"
          n153 = case shown="False" w1627 {
            selector: w1627 -> [_ w1713]
            tunnel: w1628 -> [w1711 w1714]
            tunnel: w1626 -> [w1710 w1712]
            tunnel: [w1709 w1712] -> w1623
            tunnel: [w1708 w1714] -> w1625
            tunnel: [w1707 w1713] -> w1624
            frame False {
              n154 = call "myRIO_BRig_generic_pathExists_fast_pathInput.vi"("input_error"=w1710, "input_filePath"=w1711) -> ("output_error"=w1709:errorcluster, "output_Iexist"=w1707:bool, "output_filePath"=w1708:path)  [unwired: 7 in]
            }
            frame True {
            }
          }
          n155 = case shown="False" w1696 {
            selector: w1696 -> [_ w1769]
            tunnel: w1695 -> [w1767 w1770]
            tunnel: w1694 -> [w1766 w1768]
            tunnel: [w1765 w1768] -> w1675
            tunnel: [w1764 w1770] -> w1698
            tunnel: [w1763 w1769] -> w1697
            frame False {
              n156 = call "myRIO_BRig_generic_pathExists_fast_pathInput.vi"("input_error"=w1766, "input_filePath"=w1767) -> ("output_error"=w1765:errorcluster, "output_Iexist"=w1763:bool, "output_filePath"=w1764:path)  [unwired: 7 in]
            }
            frame True {
            }
          }
          n157 = case shown="False" w1688 {
            selector: w1688 -> [_ w1761]
            tunnel: w1689 -> [w1759 w1762]
            tunnel: w1674 -> [w1758 w1760]
            tunnel: [w1757 w1760] -> w1673
            tunnel: [w1756 w1762] -> w1687
            tunnel: [w1755 w1761] -> w1686
            frame False {
              n158 = call "myRIO_BRig_generic_pathExists_fast_pathInput.vi"("input_error"=w1758, "input_filePath"=w1759) -> ("output_error"=w1757:errorcluster, "output_Iexist"=w1755:bool, "output_filePath"=w1756:path)  [unwired: 7 in]
            }
            frame True {
            }
          }
          n159 = case shown="False" w1671 {
            selector: w1671 -> [_ w1753]
            tunnel: w1672 -> [w1751 w1754]
            tunnel: w1670 -> [w1750 w1752]
            tunnel: [w1749 w1752] -> w1669
            tunnel: [w1748 w1754] -> w1667
            tunnel: [w1747 w1753] -> w1668
            frame False {
              n160 = call "myRIO_BRig_generic_pathExists_fast_pathInput.vi"("input_error"=w1750, "input_filePath"=w1751) -> ("output_error"=w1749:errorcluster, "output_Iexist"=w1747:bool, "output_filePath"=w1748:path)  [unwired: 7 in]
            }
            frame True {
            }
          }
          n161 = case shown="False" w1665 {
            selector: w1665 -> [_ w1745]
            tunnel: w1666 -> [w1743 w1746]
            tunnel: w1664 -> [w1742 w1744]
            tunnel: [w1741 w1744] -> w1663
            tunnel: [w1740 w1746] -> w1661
            tunnel: [w1739 w1745] -> w1662
            frame False {
              n162 = call "myRIO_BRig_generic_pathExists_fast_pathInput.vi"("input_error"=w1742, "input_filePath"=w1743) -> ("output_error"=w1741:errorcluster, "output_Iexist"=w1739:bool, "output_filePath"=w1740:path)  [unwired: 7 in]
            }
            frame True {
            }
          }
          n163 = case shown="False" w1659 {
            selector: w1659 -> [_ w1737]
            tunnel: w1658 -> [w1735 w1738]
            tunnel: w1660 -> [w1734 w1736]
            tunnel: [w1733 w1736] -> w1655
            tunnel: [w1732 w1738] -> w1657
            tunnel: [w1731 w1737] -> w1656
            frame False {
              n164 = call "myRIO_BRig_generic_pathExists_fast_pathInput.vi"("input_error"=w1734, "input_filePath"=w1735) -> ("output_error"=w1733:errorcluster, "output_Iexist"=w1731:bool, "output_filePath"=w1732:path)  [unwired: 7 in]
            }
            frame True {
            }
          }
          n165 = case shown="False" w1653 {
            selector: w1653 -> [_ w1729]
            tunnel: w1654 -> [w1727 w1730]
            tunnel: w1652 -> [w1726 w1728]
            tunnel: [w1725 w1728] -> w1651
            tunnel: [w1724 w1730] -> w1649
            tunnel: [w1723 w1729] -> w1650
            frame False {
              n166 = call "myRIO_BRig_generic_pathExists_fast_pathInput.vi"("input_error"=w1726, "input_filePath"=w1727) -> ("output_error"=w1725:errorcluster, "output_Iexist"=w1723:bool, "output_filePath"=w1724:path)  [unwired: 7 in]
            }
            frame True {
            }
          }
          n167 = case shown="False" w1647 {
            selector: w1647 -> [_ w1721]
            tunnel: w1648 -> [w1719 w1722]
            tunnel: w1646 -> [w1718 w1720]
            tunnel: [w1717 w1720] -> w1645
            tunnel: [w1716 w1722] -> w1643
            tunnel: [w1715 w1721] -> w1644
            frame False {
              n168 = call "myRIO_BRig_generic_pathExists_fast_pathInput.vi"("input_error"=w1718, "input_filePath"=w1719) -> ("output_error"=w1717:errorcluster, "output_Iexist"=w1715:bool, "output_filePath"=w1716:path)  [unwired: 7 in]
            }
            frame True {
            }
          }
        }
        frame #3 {
          # "Re-check\nstorage"
          n169 = Not(x=w1849) -> (.not. x?=w1856:bool)
          n170 = Not(x=w1817) -> (.not. x?=w1827:bool)
          n171 = Not(x=w1841) -> (.not. x?=w1846:bool)
          n172 = Not(x=w1815) -> (.not. x?=w1825:bool)
          n173 = Not(x=w1802) -> (.not. x?=w1823:bool)
          n174 = Not(x=w1800) -> (.not. x?=w1821:bool)
          n175 = Not(x=w1775) -> (.not. x?=w1779:bool)
          n176 = Not(x=w1798) -> (.not. x?=w1819:bool)
          n177 = And(x=w1856, y=w1855) -> (x .and. y?=w1854:bool)
          n178 = And(x=w1827, y=w1816) -> (x .and. y?=w1826:bool)
          n179 = And(x=w1846, y=w1845) -> (x .and. y?=w1842:bool)
          n180 = And(x=w1825, y=w1814) -> (x .and. y?=w1824:bool)
          n181 = And(x=w1823, y=w1801) -> (x .and. y?=w1822:bool)
          n182 = And(x=w1821, y=w1799) -> (x .and. y?=w1820:bool)
          n183 = And(x=w1779, y=w1778) -> (x .and. y?=w1773:bool)
          n184 = And(x=w1819, y=w1797) -> (x .and. y?=w1818:bool)
          n185 = case shown="True" w1854 {
            selector: w1854 -> [_ w1924]
            tunnel: w1853 -> [_ w1926]
            tunnel: w1852 -> [_ w1925]
            tunnel: w1851 -> [w1920 w1923]
            tunnel: [w1920 w1922] -> w1839
            tunnel: [w1919 w1921] -> w1850
            tunnel: w1849 -> [w1919 _]
            frame False {
            }
            frame True {
              n186 = call "myRIO_BRig_generic_pathMove_pathInput.vi"("input_error"=w1923, "input_Ioverwrite"=w1924, "input_filePath_target"=w1925, "input_filePath_source"=w1926) -> ("output_error"=w1922:errorcluster, "output_Iexist"=w1921:bool)  [unwired: 5 in, 1 out]
            }
          }
          n187 = case shown="True" w1826 {
            selector: w1826 -> [_ w1908]
            tunnel: w1808 -> [_ w1910]
            tunnel: w1805 -> [_ w1909]
            tunnel: w1810 -> [w1904 w1907]
            tunnel: [w1904 w1906] -> w1809
            tunnel: [w1903 w1905] -> w1813
            tunnel: w1817 -> [w1903 _]
            frame False {
            }
            frame True {
              n188 = call "myRIO_BRig_generic_pathMove_pathInput.vi"("input_error"=w1907, "input_Ioverwrite"=w1908, "input_filePath_target"=w1909, "input_filePath_source"=w1910) -> ("output_error"=w1906:errorcluster, "output_Iexist"=w1905:bool)  [unwired: 5 in, 1 out]
            }
          }
          n189 = case shown="True" w1842 {
            selector: w1842 -> [_ w1916]
            tunnel: w1844 -> [_ w1918]
            tunnel: w1843 -> [_ w1917]
            tunnel: w1838 -> [w1912 w1915]
            tunnel: [w1912 w1914] -> w1837
            tunnel: [w1911 w1913] -> w1840
            tunnel: w1841 -> [w1911 _]
            frame False {
            }
            frame True {
              n190 = call "myRIO_BRig_generic_pathMove_pathInput.vi"("input_error"=w1915, "input_Ioverwrite"=w1916, "input_filePath_target"=w1917, "input_filePath_source"=w1918) -> ("output_error"=w1914:errorcluster, "output_Iexist"=w1913:bool)  [unwired: 5 in, 1 out]
            }
          }
          n191 = case shown="True" w1824 {
            selector: w1824 -> [_ w1900]
            tunnel: w1807 -> [_ w1902]
            tunnel: w1806 -> [_ w1901]
            tunnel: w1804 -> [w1896 w1899]
            tunnel: [w1896 w1898] -> w1803
            tunnel: [w1895 w1897] -> w1812
            tunnel: w1815 -> [w1895 _]
            frame False {
            }
            frame True {
              n192 = call "myRIO_BRig_generic_pathMove_pathInput.vi"("input_error"=w1899, "input_Ioverwrite"=w1900, "input_filePath_target"=w1901, "input_filePath_source"=w1902) -> ("output_error"=w1898:errorcluster, "output_Iexist"=w1897:bool)  [unwired: 5 in, 1 out]
            }
          }
          n193 = case shown="True" w1822 {
            selector: w1822 -> [_ w1892]
            tunnel: w1790 -> [_ w1894]
            tunnel: w1789 -> [_ w1893]
            tunnel: w1788 -> [w1888 w1891]
            tunnel: [w1888 w1890] -> w1787
            tunnel: [w1887 w1889] -> w1786
            tunnel: w1802 -> [w1887 _]
            frame False {
            }
            frame True {
              n194 = call "myRIO_BRig_generic_pathMove_pathInput.vi"("input_error"=w1891, "input_Ioverwrite"=w1892, "input_filePath_target"=w1893, "input_filePath_source"=w1894) -> ("output_error"=w1890:errorcluster, "output_Iexist"=w1889:bool)  [unwired: 5 in, 1 out]
            }
          }
          n195 = case shown="True" w1820 {
            selector: w1820 -> [_ w1884]
            tunnel: w1793 -> [_ w1886]
            tunnel: w1792 -> [_ w1885]
            tunnel: w1791 -> [w1880 w1883]
            tunnel: [w1880 w1882] -> w1785
            tunnel: [w1879 w1881] -> w1784
            tunnel: w1800 -> [w1879 _]
            frame False {
            }
            frame True {
              n196 = call "myRIO_BRig_generic_pathMove_pathInput.vi"("input_error"=w1883, "input_Ioverwrite"=w1884, "input_filePath_target"=w1885, "input_filePath_source"=w1886) -> ("output_error"=w1882:errorcluster, "output_Iexist"=w1881:bool)  [unwired: 5 in, 1 out]
            }
          }
          n197 = case shown="True" w1773 {
            selector: w1773 -> [_ w1868]
            tunnel: w1772 -> [_ w1870]
            tunnel: w1771 -> [_ w1869]
            tunnel: w1777 -> [w1864 w1867]
            tunnel: [w1864 w1866] -> w1776
            tunnel: [w1863 w1865] -> w1774
            tunnel: w1775 -> [w1863 _]
            frame False {
            }
            frame True {
              n198 = call "myRIO_BRig_generic_pathMove_pathInput.vi"("input_error"=w1867, "input_Ioverwrite"=w1868, "input_filePath_target"=w1869, "input_filePath_source"=w1870) -> ("output_error"=w1866:errorcluster, "output_Iexist"=w1865:bool)  [unwired: 5 in, 1 out]
            }
          }
          n199 = case shown="True" w1818 {
            selector: w1818 -> [_ w1876]
            tunnel: w1796 -> [_ w1878]
            tunnel: w1795 -> [_ w1877]
            tunnel: w1794 -> [w1872 w1875]
            tunnel: [w1872 w1874] -> w1783
            tunnel: [w1871 w1873] -> w1782
            tunnel: w1798 -> [w1871 _]
            frame False {
            }
            frame True {
              n200 = call "myRIO_BRig_generic_pathMove_pathInput.vi"("input_error"=w1875, "input_Ioverwrite"=w1876, "input_filePath_target"=w1877, "input_filePath_source"=w1878) -> ("output_error"=w1874:errorcluster, "output_Iexist"=w1873:bool)  [unwired: 5 in, 1 out]
            }
          }
        }
        frame #4 {
          # "Re-check\nlabel"
          n201 = Not(x=w1971) -> (.not. x?=w1981:bool)
          n202 = Not(x=w1973) -> (.not. x?=w1982:bool)
          n203 = And(x=w1981, y=w1970) -> (x .and. y?=w1969:bool)
          n204 = And(x=w1982, y=w1972) -> (x .and. y?=w1968:bool)
          n205 = Not(x=w2014) -> (.not. x?=w2013:bool)
          n206 = Not(x=w1975) -> (.not. x?=w1983:bool)
          n207 = Not(x=w1935) -> (.not. x?=w1937:bool)
          n208 = Not(x=w1977) -> (.not. x?=w1984:bool)
          n209 = And(x=w2013, y=w2015) -> (x .and. y?=w2016:bool)
          n210 = Not(x=w2009) -> (.not. x?=w2010:bool)
          n211 = And(x=w1983, y=w1974) -> (x .and. y?=w1967:bool)
          n212 = And(x=w1937, y=w1934) -> (x .and. y?=w1936:bool)
          n213 = Not(x=w1980) -> (.not. x?=w1985:bool)
          n214 = And(x=w1984, y=w1976) -> (x .and. y?=w1966:bool)
          n215 = And(x=w2010, y=w2008) -> (x .and. y?=w2007:bool)
          n216 = And(x=w1985, y=w1979) -> (x .and. y?=w1978:bool)
          n217 = case shown="True" w2016 {
            selector: w2016 -> [_ w2113]
            tunnel: w2021 -> [_ w2112]
            tunnel: w2020 -> [w2106 w2111]
            tunnel: w2019 -> [w2105 w2110]
            tunnel: [w2105 w2108] -> w2004
            tunnel: [w2106 w2109] -> w2005
            tunnel: [w2104 w2107] -> w2017
            tunnel: w2018 -> [w2104 _]
            frame False {
            }
            frame True {
              n218 = call "myRIO_BRig_Host_formatData_getHeaders_dataBlock.vi"() -> ("output_stringArray_dataBlock"=w2114:string[])  [unwired: 11 in]
              n219 = call "myRIO_BRig_Host_formatData_test3_p2.vi"("input_headers"=w2114, "input_error"=w2110, "input_Iexist"=w2113, "input_filePath"=w2112, "input_hdl_Workbooks"=w2111) -> ("output_error"=w2108:errorcluster, "output_newFilePath"=w2107:path, "output_hdl_Worksbooks"=w2109:refnum<k7>)  [unwired: 4 in]
            }
          }
          n220 = case shown="True" w2007 {
            selector: w2007 -> [_ w2103]
            tunnel: w2006 -> [_ w2102]
            tunnel: w2005 -> [w2095 w2101]
            tunnel: w2004 -> [w2094 w2100]
            tunnel: [w2094 w2098] -> w1955
            tunnel: [w2095 w2099] -> w1954
            tunnel: [w2093 w2097] -> w2002
            tunnel: w2003 -> [w2093 _]
            frame False {
            }
            frame True {
              n221 = call "myRIO_BRig_Host_formatData_getHeaders_dataCurrent.vi"() -> ("output_stringArray_dataCurrent"=w2096:string[])  [unwired: 11 in]
              n222 = call "myRIO_BRig_Host_formatData_test3_p2.vi"("input_headers"=w2096, "input_error"=w2100, "input_Iexist"=w2103, "input_filePath"=w2102, "input_hdl_Workbooks"=w2101) -> ("output_error"=w2098:errorcluster, "output_newFilePath"=w2097:path, "output_hdl_Worksbooks"=w2099:refnum<k7>)  [unwired: 4 in]
            }
          }
          n223 = case shown="True" w1978 {
            selector: w1978 -> [_ w2092]
            tunnel: w1965 -> [_ w2091]
            tunnel: w1954 -> [w2084 w2090]
            tunnel: w1955 -> [w2083 w2089]
            tunnel: [w2083 w2087] -> w1953
            tunnel: [w2084 w2088] -> w1952
            tunnel: [w2082 w2086] -> w1945
            tunnel: w1963 -> [w2082 _]
            frame False {
            }
            frame True {
              n224 = call "myRIO_BRig_Host_formatData_getHeaders_dataExp.vi"() -> ("output_stringArray_dataExp"=w2085:string[])  [unwired: 11 in]
              n225 = call "myRIO_BRig_Host_formatData_test3_p2.vi"("input_headers"=w2085, "input_error"=w2089, "input_Iexist"=w2092, "input_filePath"=w2091, "input_hdl_Workbooks"=w2090) -> ("output_error"=w2087:errorcluster, "output_newFilePath"=w2086:path, "output_hdl_Worksbooks"=w2088:refnum<k7>)  [unwired: 4 in]
            }
          }
          n226 = case shown="True" w1966 {
            selector: w1966 -> [_ w2081]
            tunnel: w1964 -> [_ w2080]
            tunnel: w1952 -> [w2073 w2079]
            tunnel: w1953 -> [w2072 w2078]
            tunnel: [w2072 w2076] -> w1950
            tunnel: [w2073 w2077] -> w1951
            tunnel: [w2071 w2075] -> w1944
            tunnel: w1962 -> [w2071 _]
            frame False {
            }
            frame True {
              n227 = call "myRIO_BRig_Host_formatData_getHeaders_dataLC.vi"() -> ("output_stringArray_dataLC"=w2074:string[])  [unwired: 11 in]
              n228 = call "myRIO_BRig_Host_formatData_test3_p2.vi"("input_headers"=w2074, "input_error"=w2078, "input_Iexist"=w2081, "input_filePath"=w2080, "input_hdl_Workbooks"=w2079) -> ("output_error"=w2076:errorcluster, "output_newFilePath"=w2075:path, "output_hdl_Worksbooks"=w2077:refnum<k7>)  [unwired: 4 in]
            }
          }
          n229 = case shown="True" w1967 {
            selector: w1967 -> [_ w2070]
            tunnel: w1960 -> [_ w2069]
            tunnel: w1951 -> [w2062 w2068]
            tunnel: w1950 -> [w2061 w2067]
            tunnel: [w2061 w2065] -> w1948
            tunnel: [w2062 w2066] -> w1949
            tunnel: [w2060 w2064] -> w1943
            tunnel: w1961 -> [w2060 _]
            frame False {
            }
            frame True {
              n230 = call "myRIO_BRig_Host_formatData_getHeaders_dataLick.vi"() -> ("output_stringArray_dataLick"=w2063:string[])  [unwired: 11 in]
              n231 = call "myRIO_BRig_Host_formatData_test3_p2.vi"("input_headers"=w2063, "input_error"=w2067, "input_Iexist"=w2070, "input_filePath"=w2069, "input_hdl_Workbooks"=w2068) -> ("output_error"=w2065:errorcluster, "output_newFilePath"=w2064:path, "output_hdl_Worksbooks"=w2066:refnum<k7>)  [unwired: 4 in]
            }
          }
          n232 = case shown="True" w1968 {
            selector: w1968 -> [_ w2059]
            tunnel: w1959 -> [_ w2058]
            tunnel: w1949 -> [w2051 w2057]
            tunnel: w1948 -> [w2050 w2056]
            tunnel: [w2050 w2054] -> w1946
            tunnel: [w2051 w2055] -> w1947
            tunnel: [w2049 w2053] -> w1942
            tunnel: w1958 -> [w2049 _]
            frame False {
            }
            frame True {
              n233 = call "myRIO_BRig_Host_formatData_getHeaders_dataMTrig.vi"() -> ("output_stringArray_dataMTrig"=w2052:string[])  [unwired: 11 in]
              n234 = call "myRIO_BRig_Host_formatData_test3_p2.vi"("input_headers"=w2052, "input_error"=w2056, "input_Iexist"=w2059, "input_filePath"=w2058, "input_hdl_Workbooks"=w2057) -> ("output_error"=w2054:errorcluster, "output_newFilePath"=w2053:path, "output_hdl_Worksbooks"=w2055:refnum<k7>)  [unwired: 4 in]
            }
          }
          n235 = case shown="True" w1969 {
            selector: w1969 -> [_ w2048]
            tunnel: w1957 -> [_ w2047]
            tunnel: w1947 -> [w2040 w2046]
            tunnel: w1946 -> [w2039 w2045]
            tunnel: [w2039 w2043] -> w1932
            tunnel: [w2040 w2044] -> w1931
            tunnel: [w2038 w2042] -> w1941
            tunnel: w1956 -> [w2038 _]
            frame False {
            }
            frame True {
              n236 = call "myRIO_BRig_Host_formatData_getHeaders_dataTrial.vi"() -> ("output_stringArray_dataTrial"=w2041:string[])  [unwired: 11 in]
              n237 = call "myRIO_BRig_Host_formatData_test3_p2.vi"("input_headers"=w2041, "input_error"=w2045, "input_Iexist"=w2048, "input_filePath"=w2047, "input_hdl_Workbooks"=w2046) -> ("output_error"=w2043:errorcluster, "output_newFilePath"=w2042:path, "output_hdl_Worksbooks"=w2044:refnum<k7>)  [unwired: 4 in]
            }
          }
          n238 = case shown="True" w1936 {
            selector: w1936 -> [_ w2037]
            tunnel: w1933 -> [_ w2036]
            tunnel: w1931 -> [w2029 w2035]
            tunnel: w1932 -> [w2028 w2034]
            tunnel: [w2028 w2032] -> w1927
            tunnel: [w2029 w2033] -> w1928
            tunnel: [w2027 w2031] -> w1929
            tunnel: w1930 -> [w2027 _]
            frame False {
            }
            frame True {
              n239 = call "myRIO_BRig_Host_formatData_getHeaders_dataAnalog.vi"() -> ("output_stringArray_dataAnalog"=w2030:string[])  [unwired: 11 in]
              n240 = call "myRIO_BRig_Host_formatData_test3_p2.vi"("input_headers"=w2030, "input_error"=w2034, "input_Iexist"=w2037, "input_filePath"=w2036, "input_hdl_Workbooks"=w2035) -> ("output_error"=w2032:errorcluster, "output_newFilePath"=w2031:path, "output_hdl_Worksbooks"=w2033:refnum<k7>)  [unwired: 4 in]
            }
          }
        }
        frame #5 {
          # "Re-check\nlabel\npart2"
          n241 = Not(x=w2145) -> (.not. x?=w2150:bool)
          n242 = Not(x=w2118) -> (.not. x?=w2120:bool)
          n243 = Not(x=w2149) -> (.not. x?=w2154:bool)
          n244 = Not(x=w2146) -> (.not. x?=w2151:bool)
          n245 = Not(x=w2148) -> (.not. x?=w2153:bool)
          n246 = Not(x=w2180) -> (.not. x?=w2181:bool)
          n247 = Not(x=w2147) -> (.not. x?=w2152:bool)
          n248 = Not(x=w2187) -> (.not. x?=w2190:bool)
          n249 = case shown="True" w2150 {
            tunnel: w2139 -> [w2205 w2210]
            tunnel: w2140 -> [_ w2209]
            tunnel: [w2205 w2208] -> w2125
            tunnel: [w2206 w2207] -> w2126
            tunnel: w2145 -> [w2206 _]
            frame False {
            }
            frame True {
              n250 = call "myRIO_BRig_generic_pathExists_fast_pathInput.vi"("input_error"=w2210, "input_filePath"=w2209) -> ("output_error"=w2208:errorcluster, "output_Iexist"=w2207:bool)  [unwired: 7 in, 1 out]
            }
          }
          n251 = case shown="True" w2120 {
            tunnel: w2116 -> [w2199 w2204]
            tunnel: w2119 -> [_ w2203]
            tunnel: [w2199 w2202] -> w2115
            tunnel: [w2200 w2201] -> w2117
            tunnel: w2118 -> [w2200 _]
            frame False {
            }
            frame True {
              n252 = call "myRIO_BRig_generic_pathExists_fast_pathInput.vi"("input_error"=w2204, "input_filePath"=w2203) -> ("output_error"=w2202:errorcluster, "output_Iexist"=w2201:bool)  [unwired: 7 in, 1 out]
            }
          }
          n253 = case shown="True" w2154 {
            tunnel: w2135 -> [w2229 w2234]
            tunnel: w2144 -> [_ w2233]
            tunnel: [w2229 w2232] -> w2133
            tunnel: [w2230 w2231] -> w2134
            tunnel: w2149 -> [w2230 _]
            frame False {
            }
            frame True {
              n254 = call "myRIO_BRig_generic_pathExists_fast_pathInput.vi"("input_error"=w2234, "input_filePath"=w2233) -> ("output_error"=w2232:errorcluster, "output_Iexist"=w2231:bool)  [unwired: 7 in, 1 out]
            }
          }
          n255 = case shown="True" w2151 {
            tunnel: w2138 -> [w2211 w2216]
            tunnel: w2141 -> [_ w2215]
            tunnel: [w2211 w2214] -> w2127
            tunnel: [w2212 w2213] -> w2128
            tunnel: w2146 -> [w2212 _]
            frame False {
            }
            frame True {
              n256 = call "myRIO_BRig_generic_pathExists_fast_pathInput.vi"("input_error"=w2216, "input_filePath"=w2215) -> ("output_error"=w2214:errorcluster, "output_Iexist"=w2213:bool)  [unwired: 7 in, 1 out]
            }
          }
          n257 = case shown="True" w2153 {
            tunnel: w2136 -> [w2223 w2228]
            tunnel: w2143 -> [_ w2227]
            tunnel: [w2223 w2226] -> w2131
            tunnel: [w2224 w2225] -> w2132
            tunnel: w2148 -> [w2224 _]
            frame False {
            }
            frame True {
              n258 = call "myRIO_BRig_generic_pathExists_fast_pathInput.vi"("input_error"=w2228, "input_filePath"=w2227) -> ("output_error"=w2226:errorcluster, "output_Iexist"=w2225:bool)  [unwired: 7 in, 1 out]
            }
          }
          n259 = case shown="True" w2181 {
            tunnel: w2156 -> [w2235 w2240]
            tunnel: w2179 -> [_ w2239]
            tunnel: [w2235 w2238] -> w2155
            tunnel: [w2236 w2237] -> w2178
            tunnel: w2180 -> [w2236 _]
            frame False {
            }
            frame True {
              n260 = call "myRIO_BRig_generic_pathExists_fast_pathInput.vi"("input_error"=w2240, "input_filePath"=w2239) -> ("output_error"=w2238:errorcluster, "output_Iexist"=w2237:bool)  [unwired: 7 in, 1 out]
            }
          }
          n261 = case shown="True" w2152 {
            tunnel: w2137 -> [w2217 w2222]
            tunnel: w2142 -> [_ w2221]
            tunnel: [w2217 w2220] -> w2129
            tunnel: [w2218 w2219] -> w2130
            tunnel: w2147 -> [w2218 _]
            frame False {
            }
            frame True {
              n262 = call "myRIO_BRig_generic_pathExists_fast_pathInput.vi"("input_error"=w2222, "input_filePath"=w2221) -> ("output_error"=w2220:errorcluster, "output_Iexist"=w2219:bool)  [unwired: 7 in, 1 out]
            }
          }
          n263 = case shown="True" w2190 {
            tunnel: w2186 -> [w2241 w2246]
            tunnel: w2189 -> [_ w2245]
            tunnel: [w2241 w2244] -> w2157
            tunnel: [w2242 w2243] -> w2188
            tunnel: w2187 -> [w2242 _]
            frame False {
            }
            frame True {
              n264 = call "myRIO_BRig_generic_pathExists_fast_pathInput.vi"("input_error"=w2246, "input_filePath"=w2245) -> ("output_error"=w2244:errorcluster, "output_Iexist"=w2243:bool)  [unwired: 7 in, 1 out]
            }
          }
        }
      }
      n265 = Merge Errors(w1086, w1087, w1089, w1088, w1084, w1083, w1082, w1030) -> (w1085:errorcluster)
    }
  }
  "error1" <- w333
  n266 = Boolean To (0,1)(Boolean=w61) -> (0, 1=w78:i16)
  n267 = Boolean To (0,1)(Boolean=w62) -> (0, 1=w77:i16)
  n268 = Boolean To (0,1)(Boolean=w63) -> (0, 1=w76:i16)
  n269 = Boolean To (0,1)(Boolean=w329) -> (0, 1=w326:i16)
  n270 = Boolean To (0,1)(Boolean=w328) -> (0, 1=w325:i16)
  n271 = Boolean To (0,1)(Boolean=w327) -> (0, 1=w324:i16)
  n272 = Boolean To (0,1)(Boolean=w52) -> (0, 1=w96:i16)
  n273 = Boolean To (0,1)(Boolean=w53) -> (0, 1=w95:i16)
  n274 = Boolean To (0,1)(Boolean=w54) -> (0, 1=w94:i16)
  n275 = Boolean To (0,1)(Boolean=w285) -> (0, 1=w291:i16)
  n276 = Boolean To (0,1)(Boolean=w284) -> (0, 1=w290:i16)
  n277 = Boolean To (0,1)(Boolean=w283) -> (0, 1=w289:i16)
  n278 = Boolean To (0,1)(Boolean=w55) -> (0, 1=w90:i16)
  n279 = Boolean To (0,1)(Boolean=w56) -> (0, 1=w89:i16)
  n280 = Boolean To (0,1)(Boolean=w57) -> (0, 1=w88:i16)
  n281 = Boolean To (0,1)(Boolean=w58) -> (0, 1=w84:i16)
  n282 = Boolean To (0,1)(Boolean=w59) -> (0, 1=w83:i16)
  n283 = Boolean To (0,1)(Boolean=w60) -> (0, 1=w82:i16)
  n284 = Boolean To (0,1)(Boolean=w66) -> (0, 1=w72:i16)
  n285 = Boolean To (0,1)(Boolean=w65) -> (0, 1=w71:i16)
  n286 = Boolean To (0,1)(Boolean=w64) -> (0, 1=w70:i16)
  n287 = Boolean To (0,1)(Boolean=w5) -> (0, 1=w11:i16)
  n288 = Boolean To (0,1)(Boolean=w4) -> (0, 1=w10:i16)
  n289 = Boolean To (0,1)(Boolean=w3) -> (0, 1=w9:i16)
  n290 = Compound Arithmetic op=ADD(w78, w77, w76) -> (w75:i16)
  n291 = case shown="3" w75 {
    tunnel: ["!!!  Error - Missing  !!!" "! Error - Saving !" "Error - Labelling" "Success"] -> w74
    frame 0, Default {
    }
    frame 1 {
    }
    frame 2 {
    }
    frame 3 {
    }
  }
  n292 = Compound Arithmetic op=ADD(w326, w325, w324) -> (w323:i16)
  n293 = case shown="3" w323 {
    tunnel: ["!!!  Error - Missing  !!!" "! Error - Saving !" "Error - Labelling" "Success"] -> w322
    frame 0, Default {
    }
    frame 1 {
    }
    frame 2 {
    }
    frame 3 {
    }
  }
  n294 = Compound Arithmetic op=ADD(w96, w95, w94) -> (w93:i16)
  n295 = case shown="3" w93 {
    tunnel: ["!!!  Error - Missing  !!!" "! Error - Saving !" "Error - Labelling" "Success"] -> w92
    frame 0, Default {
    }
    frame 1 {
    }
    frame 2 {
    }
    frame 3 {
    }
  }
  n296 = Compound Arithmetic op=ADD(w291, w290, w289) -> (w288:i16)
  n297 = case shown="3" w288 {
    tunnel: ["!!!  Error - Missing  !!!" "! Error - Saving !" "Error - Labelling" "Success"] -> w287
    frame 0, Default {
    }
    frame 1 {
    }
    frame 2 {
    }
    frame 3 {
    }
  }
  n298 = Compound Arithmetic op=ADD(w90, w89, w88) -> (w87:i16)
  n299 = case shown="3" w87 {
    tunnel: ["!!!  Error - Missing  !!!" "! Error - Saving !" "Error - Labelling" "Success"] -> w86
    frame 0, Default {
    }
    frame 1 {
    }
    frame 2 {
    }
    frame 3 {
    }
  }
  n300 = Compound Arithmetic op=ADD(w84, w83, w82) -> (w81:i16)
  n301 = case shown="3" w81 {
    tunnel: ["!!!  Error - Missing  !!!" "! Error - Saving !" "Error - Labelling" "Success"] -> w80
    frame 0, Default {
    }
    frame 1 {
    }
    frame 2 {
    }
    frame 3 {
    }
  }
  n302 = Compound Arithmetic op=ADD(w72, w71, w70) -> (w69:i16)
  n303 = case shown="3" w69 {
    tunnel: ["!!!  Error - Missing  !!!" "! Error - Saving !" "Error - Labelling" "Success"] -> w68
    frame 0, Default {
    }
    frame 1 {
    }
    frame 2 {
    }
    frame 3 {
    }
  }
  n304 = Compound Arithmetic op=ADD(w11, w10, w9) -> (w8:i16)
  n305 = case shown="3" w8 {
    tunnel: ["!!!  Error - Missing  !!!" "! Error - Saving !" "Error - Labelling" "Success"] -> w7
    frame 0, Default {
    }
    frame 1 {
    }
    frame 2 {
    }
    frame 3 {
    }
  }
  n306 = case shown="False" w338 {
    tunnel: w339 -> [w2282 w2288]
    tunnel: w341 -> [w2281 w2286]
    tunnel: [w2285 w2288] -> w334
    tunnel: [w2284 w2287] -> w336
    tunnel: w340 -> [w2280 w2287]
    tunnel: [w2279 w2286] -> w337
    frame False {
      n307 = invoke class="Workbooks" method="Close"(reference=w2281, error in=w2282) -> (reference out=w2279:refnum<k7>, error out=w2283:errorcluster)  [unwired: 1 in, 1 out]
      n308 = invoke class="_Application" method="Quit"(reference=w2280, error in=w2283) -> (reference out=w2284:refnum<k7>, error out=w2285:errorcluster)  [unwired: 1 in, 1 out]
    }
    frame True {
    }
  }
  n309 = Concatenate Strings("DataMTrig = ", w74) -> (w48:string)
  n310 = Concatenate Strings("DataBlock = ", w322) -> (w282:string)
  n311 = Concatenate Strings("DataExp = ", w92) -> (w51:string)
  n312 = Concatenate Strings("DataCurrent = ", w287) -> (w281:string)
  n313 = Concatenate Strings("DataLC = ", w86) -> (w50:string)
  n314 = Concatenate Strings("DataLick = ", w80) -> (w49:string)
  n315 = Concatenate Strings("DataTrial = ", w68) -> (w47:string)
  n316 = Concatenate Strings("DataAnalog = ", w7) -> (w1:string)
  n317 = Concatenate Strings(w282, w2, w281, w2, w51, w2, w50, w2, w49, w2, w48, w2, w47, w2, w1) -> (w280:string)
  n318 = flat-sequence {
    tunnel: w280 -> [w2290]
    tunnel: [w2289] -> w98
    tunnel: w97 -> [w2289]
    frame #0 {
      n319 = One Button Dialog(message=w2290) -> ()  [unwired: 1 in, 1 out]
    }
  }
  n320 = Close Reference(reference=w337, error in (no error)=w334) -> (error out=w335:errorcluster)
  n321 = Unbundle By Name(w98) -> ("code"=w332:i32)
  n322 = Close Reference(reference=w336, error in (no error)=w335) -> (error out=w97:errorcluster)
  "error2" <- w97
  n323 = Equal?(x=w332, y=-2146827284) -> (x = y?=w330:bool)
  n324 = case shown="True" w330 {
    frame False {
    }
    frame True {
      n325 = One Button Dialog(message="Use \"Alt-Ctrl-Delete\" to close Excel") -> ()  [unwired: 1 in, 1 out]
    }
  }
